vi "FL24 Washer Tool Main.vi"() -> ()   [LabVIEW 2016]
uses:
  Common/LabVIEW GEA2 Toolkit/LabVIEW_GEA2_Toolkit.lvlibp/type defs/Data In.ctl
  Common/LabVIEW GEA2 Toolkit/LabVIEW_GEA2_Toolkit.lvlibp/type defs/Source_Destination.ctl
  Common/LabVIEW GEA2 Toolkit/LabVIEW_GEA2_Toolkit.lvlibp/type defs/Data Type.ctl
  Common/LabVIEW GEA2 Toolkit/LabVIEW_GEA2_Toolkit.lvlibp/type defs/ERD Read Data In.ctl
  Laundry Tool 2.0 Support/type defs2/Select _Graph_Brass.ctl
  Laundry Tool 1.0 Support/type defs/ERD_Graph_All.ctl
  Laundry Tool 1.0 Support/type defs/ERD_Graph.ctl
  Laundry Tool 1.0 Support/type defs/Version.ctl
  Laundry Tool 2.0 Support/type defs2/ERD_Always_Show_FL24_Washer.ctl
  Laundry Tool 1.0 Support/type defs/Fault_Buffer_Status.ctl
  Laundry Tool 2.0 Support/type defs2/Diagnostics_Table.ctl
  Laundry Tool 1.0 Support/type defs/Cycle_Diag_Buffer_Status.ctl
  Laundry Tool 2.0 Support/type defs2/ERD_Data_Loop_Control_Brass.ctl
  Laundry Tool 2.0 Support/type defs2/ERD_Loop_States_Brass.ctl
  Laundry Tool 2.0 Support/type defs2/Error_Command_Brass.ctl
  Laundry Tool 2.0 Support/type defs2/DAQ_States_Brass.ctl
  Common/GExplorer Support/typedefs/GExplorer_Data_Cluster.ctl
  Laundry Tool 1.0 Support/type defs/Cont_Send_States.ctl
  Laundry Tool 2.0 Support/type defs2/Cont_Send_States_Brass.ctl
  Common/LabVIEW GEA2 Toolkit/LabVIEW_GEA2_Toolkit.lvlibp/type defs/Data Out.ctl
  Common/LabVIEW GEA2 Toolkit/LabVIEW_GEA2_Toolkit.lvlibp/type defs/ERD Write Data In.ctl
  Laundry Tool 2.0 Support/type defs2/DAQ_Control_Command_Brass.ctl
  Laundry Tool 2.0 Support/type defs2/ERD_Loop_Control_Command_Brass.ctl
  Laundry Tool 2.0 Support/type defs2/GEA2_Control_Command_Brass.ctl
  <vilib>/DAQmx/read.llb/DAQmx Read (Digital 1D Bool NChan 1Samp 1Line).vi
  <vilib>/DAQmx/read.llb/DAQmx Read (Digital 1D U8 1Chan NSamp).vi
  <vilib>/DAQmx/write.llb/DAQmx Write (Digital Bool 1Line 1Point).vi
  <vilib>/DAQmx/read.llb/DAQmx Read (Counter U32 1Chan 1Samp).vi
  <vilib>/DAQmx/write.llb/DAQmx Write (Analog 1D DBL NChan 1Samp).vi
  <vilib>/DAQmx/write.llb/DAQmx Write (Digital 1D Bool NChan 1Samp 1Line).vi
  Common/LabVIEW GEA2 Toolkit/LabVIEW_GEA2_Toolkit.lvlibp/advanced/GEA2 Message Received Event Handler.vi
  <vilib>/DAQmx/create/channels.llb/DAQmx Create Channel (DO-Digital Output).vi
  <vilib>/DAQmx/create/channels.llb/DAQmx Create Channel (DI-Digital Input).vi
  <vilib>/DAQmx/configure/timing.llb/DAQmx Timing (Sample Clock).vi
  <vilib>/DAQmx/create/channels.llb/DAQmx Create Channel (CO-Pulse Generation-Frequency).vi
  <vilib>/DAQmx/configure/timing.llb/DAQmx Timing (Implicit).vi
  <vilib>/DAQmx/create/channels.llb/DAQmx Create Channel (CI-Count Edges).vi
  <vilib>/DAQmx/create/channels.llb/DAQmx Create Channel (AO-Voltage-Basic).vi
  <vilib>/DAQmx/miscellaneous.llb/DAQmx Fill In Error Info.vi
  C:/Automation/DLLs/PC Dot Net/GeaCommunication.dll
  Common/LabVIEW GEA2 Toolkit/LabVIEW_GEA2_Toolkit.lvlibp
  Automation/Product Specific/Clothes Care/2015 VA Washer/Projects/2015 VA Washer.lvlib
  <resource>/objmgr/daqmx.rc
panel:
  in  "Data ON":bool=TRUE
  out "ERD_Always Show":T1
  in  "Stop":bool
  out "Fault Status":bool
  out "Log Rate (ms)":u32
  in  "Tab Control":T2(tab)
  in  "Filter Data":bool=TRUE
  in  "Start Send":bool
  in  "Cmd":string
  in  "Filter Log":bool
  in  "Msg Rate (ms)":u32=1000 min=50 step=50
  out "CSV File Log Path":path=path "C:/Users/502129737/Desktop/1"
  in  "Clear":bool
  out "GEA2 Log":string
  in  "Board Index":u8 max=0 step=1
  out "Board ID":string="0"
  in  "GEA2 Send":T3={"Source"=228, "Destination"=52, "Command"=0, "Message"=""} {"Command" format="%02x"; "Destination" format="%02x"; "Source" format="%02x"}
  in  "Send Button":bool
  in  "GEA2 Log Length":i32=100000
  in  "Save Log":bool
  out "Version":T4
  in  "GEA Inputs":T5={"Source"=228, "Destination"=52} {"Destination" format="%.0x"; "Source" format="%.0x"}
  in  "Read ERD List":T6[](array[typedef])=[{"ERD Number"=0, "Data Type"=enum."string"}] {"ERD Number" format="%.0x"}
  out "Read ERD Data Out":cluster{"ERD Number":u16, "Data":string}[](array[cluster]) {"ERD Number" format="%.0x"}
  in  "Read ERD":bool
  in  "Write ERD":bool
  in  "Write ERD List":T8(array[cluster])=[{"ERD Number"=0, "Data Type"=enum."string", "Data"=""}] {"ERD Number" format="%.0x"}
  out "All Loads":u16[][](graph)=[[0, 100, 200, 300, 400]]
  in  "ERD Graphing ON":bool
  out "ERD Graph  Ind":T9
  in  "ERD Graph Cntrl":T10={"ERD 3"={"ERD #"=62250, "Data Type"=enum."uint16_t", "Scaler"=32}, "ERD 2"={"ERD #"=62250, "Data Type"=enum."uint16_t", "Scaler"=32}, "ERD 1"={"ERD #"=62250, "Data Type"=enum."uint16_t", "Scaler"=32}} {"ERD 1"."Scaler" min=1; "ERD 1"."ERD #" format="%.0x"; "ERD 2"."Scaler" min=1; "ERD 2"."ERD #" format="%.0x"; "ERD 3"."Scaler" min=1; "ERD 3"."ERD #" format="%.0x"}
  in  "Graphing ON":bool=TRUE
  in  "Select Graph":T12
  out "ERD 3":dbl(graph)
  out "ERD 2":dbl(graph)
  out "ERD 1":dbl(graph)
  in  "Save Fault Log":bool
  in  "Clear Fault Table Buffer":bool
  in  "Clear Fault Seq Buffer":bool
  in  "Fault ON":bool
  out "Fault Table Buffer":string[][](table)
  out "Fault Sequence Buffer":string
  out "Seq Buffer Status":T13
  out "Table Buffer Status":T13
  in  "Save Cycle History Log":bool
  in  "Clear Cycle Buffer":bool
  out "Cycle Buffer Status":T14
  in  "Get Cycle History":bool
  out "Diagnostics Table":T15
  in  "Test Mode":cluster{"Exit":bool, "Enter":bool}
  in  "Lid Lock":cluster{"Lock Lid":bool, "Unlock Lid":bool}
  in  "HE/LE ?":enum16{"HE", "LE"}(ring)
  in  "LL (M - A)":bool=TRUE
  in  "Lid Lock Feedback":bool
  in  "MS (M - A)":bool=TRUE
  out "DAQ Status":string
  out "Drain Pump":bool
  out "Mode Shift":bool
  out "Recirc Pump":bool
  out "Cold Valve":bool
  out "Hot Valve":bool
  out "Spray/Rinse Valve":bool
  out "Fabric SoftValve":bool
  in  "AC Power":bool=TRUE
  in  "Mode Shift FB":bool
  in  "Lid Status":bool=TRUE
  in  "Pressure":dbl(slide) min=0.0 max=5.0 step=0.5 scale=0.0..5.0 scale format="%#_3g"
  in  "Motor Current":dbl(slide)=2.5 min=0.0 max=5.0 step=0.5 scale=0.0..5.0 scale format="%#_3g"
  in  "Turn On DAQ":bool
  out "DAQ On?":bool
  in  "Basket RPM":dbl=1.0 min=1.0 max=800.0 step=5.0
  in  "Temperature":dbl(slide)=2.5 min=0.0 max=5.0 step=0.5 scale=0.0..5.0 scale format="%#_3g"
  out "Triac CW":bool
  out "Traic CCW":bool
  out "CCW":u32
  out "CW":u32
  in  "ERD Read List":T16(array[cluster])=[{"Boolean"=TRUE, "ERD Number"=1, "ERD Name"="Model Number", "Data Type"=enum."string"}, {"Boolean"=TRUE, "ERD Number"=2, "ERD Name"="Serial Number", "Data Type"=enum."string"}, {"Boolean"=TRUE, "ERD Number"=8192, "ERD Name"="Machine Status", "Data Type"=enum."uint8_t"}, {"Boolean"=TRUE, "ERD Number"=8202, "ERD Name"="Cycle Name", "Data Type"=enum."string"}, {"Boolean"=TRUE, "ERD Number"=8213, "ERD Name"="Soil Level", "Data Type"=enum."string"}, {"Boolean"=TRUE, "ERD Number"=142, "ERD Name"="Cycle Count", "Data Type"=enum."uint32_t"}, {"Boolean"=TRUE, "ERD Number"=8193, "ERD Name"="Sub-Cycle", "Data Type"=enum."string"}, {"Boolean"=TRUE, "ERD Number"=141, "ERD Name"="System Runtime", "Data Type"=enum."uint32_t"}, {"Boolean"=TRUE, "ERD Number"=8208, "ERD Name"="Delay Time", "Data Type"=enum."uint16_t"}, {"Boolean"=FALSE, "ERD Number"=256, "ERD Name"="Version", "Data Type"=enum."string"}, {"Boolean"=TRUE, "ERD Number"=70, "ERD Name"="Cycle Time", "Data Type"=enum."uint16_t"}, {"Boolean"=TRUE, "ERD Number"=8206, "ERD Name"="Operating Mode", "Data Type"=enum."string"}, {"Boolean"=TRUE, "ERD Number"=8214, "ERD Name"="Temp Level", "Data Type"=enum."uint8_t"}, {"Boolean"=TRUE, "ERD Number"=8215, "ERD Name"="Spin Level", "Data Type"=enum."uint8_t"}, {"Boolean"=TRUE, "ERD Number"=61440, "ERD Name"="Water Level", "Data Type"=enum."uint8_t"}, {"Boolean"=TRUE, "ERD Number"=8216, "ERD Name"="Rinse Option", "Data Type"=enum."uint8_t"}, {"Boolean"=TRUE, "ERD Number"=8236, "ERD Name"="Basket Speed", "Data Type"=enum."uint16_t"}, {"Boolean"=TRUE, "ERD Number"=61451, "ERD Name"="Loads 2", "Data Type"=enum."uint8_t"}, {"Boolean"=TRUE, "ERD Number"=8210, "ERD Name"="Door Status", "Data Type"=enum."string"}, {"Boolean"=TRUE, "ERD Number"=8211, "ERD Name"="Lock Status", "Data Type"=enum."string"}] {"ERD Number" format="%.0x"}
  out "Error Out":errorcluster
  in  "Error In":errorcluster
  # "Software Version"
  # "UI"
  # "MC"
  # "Must input a valid ERD# and Data Type\nDO NOT Leave Blank \nIf no scaler use value of 01"
  # "Contact:\n\nDerek Hibdon\nderek.hibdon@ge.com"
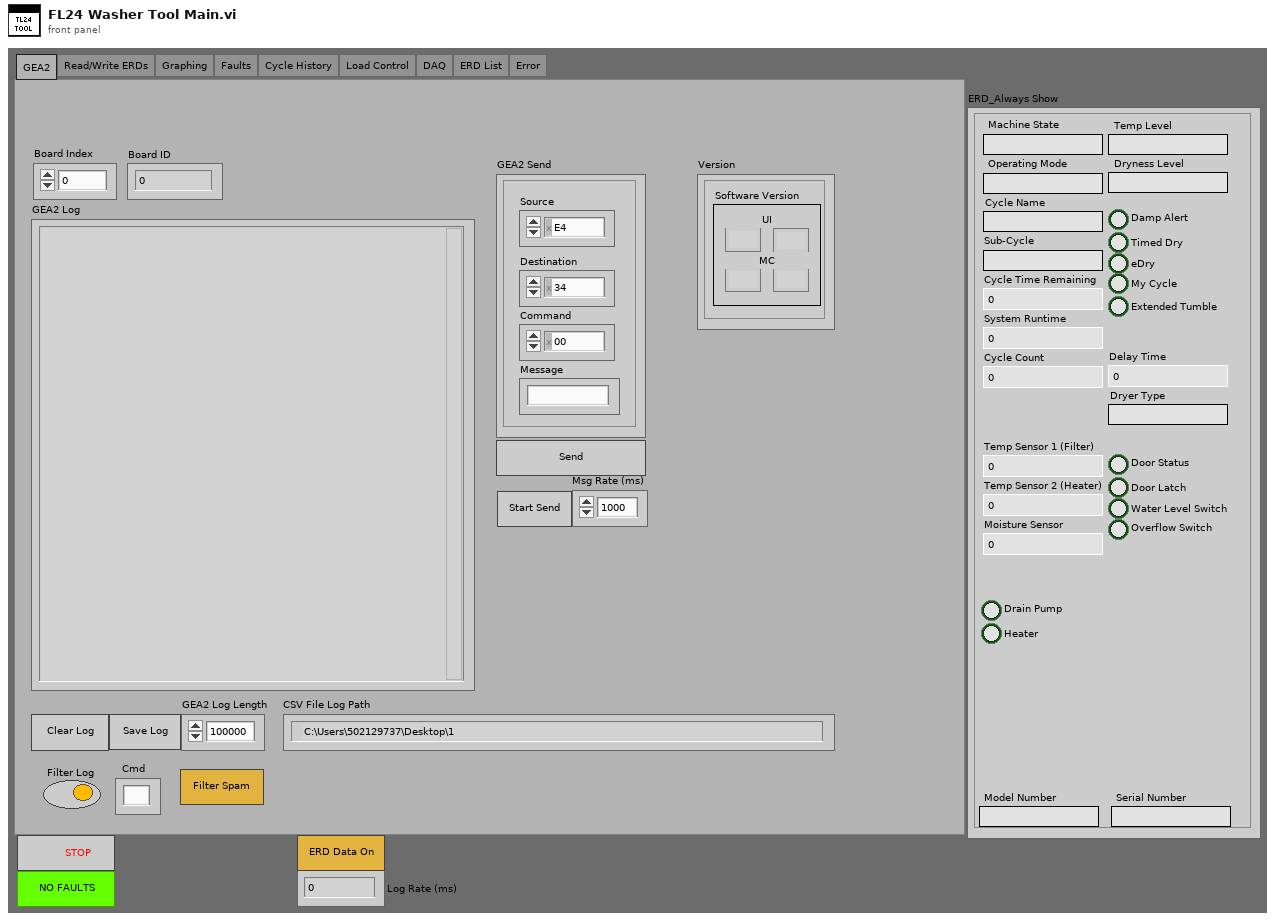
[diagram p1: front panel]
types:
  T1 = typedef "ERD_Always_Show_FL24_Washer.ctl" = cluster{"Machine State":string, "Cycle Count":u32, "Dryness Level":string, "Temp Level":string, "Delay Time":u16, "Sub-Cycle":string, "Cycle Name":string, "Model Number":string, "Serial Number":string, "System Runtime":u32, "Cycle Time Remaining":u16, "Operating Mode":string, "Temp Sensor 1 (Filter)":u16, "Drain Pump":bool, "Water Level Switch":bool, "Overflow Switch":bool, "Door Status":bool, "Door Latch":bool, "Heater":bool, "Temp Sensor 2 (Heater)":u16, "Moisture Sensor":u16, "Dryer Type":string, "eDry":bool, "Damp Alert":bool, "Timed Dry":bool, "My Cycle":bool, "Extended Tumble":bool}
  T2 = enum32{"GEA2", "Read/Write ERDs", "Graphing", "Faults", "Cycle History", "Load Control", "DAQ", "ERD List", "Error"}
  T3 = typedef "LabVIEW_GEA2_Toolkit.lvlibp/Data In.ctl" = cluster{"Source":u8, "Destination":u8, "Command":u8, "Message":string}
  T4 = typedef "Version.ctl" = cluster{"Critical Major":string, "Critical Minor":string, "Non-Critical Minor":string, "Non-Critical Major":string}
  T5 = typedef "LabVIEW_GEA2_Toolkit.lvlibp/Source_Destination.ctl" = cluster{"Source":u8, "Destination":u8}
  T6 = typedef "LabVIEW_GEA2_Toolkit.lvlibp/ERD Read Data In.ctl" = cluster{"ERD Number":u16, "Data Type":T7}
  T7 = typedef "LabVIEW_GEA2_Toolkit.lvlibp/Data Type.ctl" = enum16{"string", "boolean", "uint8_t", "uint16_t", "uint32_t", "uint64_t", "int8_t", "int16_t", "int32_t", "int64_t"}
  T8 = cluster{"ERD Number":u16, "Data Type":T7, "Data":string}[]
  T9 = cluster{"ERD Value 1":dbl, "ERD Value 2":dbl, "ERD Value 3":dbl}
  T10 = typedef "ERD_Graph_All.ctl" = cluster{"ERD 3":T11, "ERD 2":T11, "ERD 1":T11}
  T11 = typedef "ERD_Graph.ctl" = cluster{"ERD #":u16, "Data Type":T7, "Scaler":u32}
  T12 = typedef "Select _Graph_Brass.ctl" = enum16{"All Loads", "ERD 1", "ERD 2", "ERD 3", "Temperature (F)", "Basket Speed (RPM)", "Tub Volume (Gal)", "Pressure (in H2O)", "Current RMS (Amps)"}
  T13 = typedef "Fault_Buffer_Status.ctl" = cluster{"Current Index":u16, "Count":u16, "Overwrite Count":u16}
  T14 = typedef "Cycle_Diag_Buffer_Status.ctl" = cluster{"Current Index":u16, "Count":u16, "Overwrite Count":u16}
  T15 = typedef "Diagnostics_Table.ctl" = string[][]
  T16 = cluster{"Boolean":bool, "ERD Number":u16, "ERD Name":string, "Data Type":enum16{"string", "boolean", "uint8_t", "uint16_t", "uint32_t", "uint64_t"}}[]
  T17 = typedef "Cont_Send_States_Brass.ctl" = enum16{"Run", "Shutdown"}
  T18 = typedef "Cont_Send_States.ctl" = enum16{"Run", "Shutdown"}
  T19 = typedef "GExplorer_Data_Cluster.ctl" = cluster{"Data":variant, "State":enum16{"Add to Log", "Clear", "Shutdown"}}
  T20 = typedef "DAQ_States_Brass.ctl" = enum16{"Wait for Init", "Rename Devices", "Verify Hardware", "Initialize", "Run", "Shutdown", "Exit"}
  T21 = typedef "ERD_Data_Loop_Control_Brass.ctl" = cluster{"Data":variant, "State":T22}
  T22 = typedef "ERD_Loop_States_Brass.ctl" = enum16{"Init", "Build ERD Read List", "Read ERDs", "Update UI", "Update Graphs", "Read Faults", "Log Data", "Pause", "Shutdown"}
  T23 = typedef "Error_Command_Brass.ctl" = enum16{"Initialize", "Handle Errors", "Report Errors"}
  T24 = typedef "LabVIEW_GEA2_Toolkit.lvlibp/ERD Write Data In.ctl" = cluster{"ERD Number":u16, "Data Type":T7, "Data":string}
  T25 = typedef "GEA2_Control_Command_Brass.ctl" = enum16{"Initialize", "Shutdown"}
  T26 = typedef "ERD_Loop_Control_Command_Brass.ctl" = enum16{"Initialize", "Shutdown"}
  T27 = typedef "DAQ_Control_Command_Brass.ctl" = enum16{"Initialize", "Shutdown", "Exit"}
  T28 = enum8{"Enabled", "Disabled", "Disabled and Grayed Out"}
  T29 = typedef "LabVIEW_GEA2_Toolkit.lvlibp/Data Out.ctl" = cluster{"Source":u8, "Destination":u8, "Command":u8, "Length":u8, "CRC":u16, "Message":string}
  T30 = typedef "LabVIEW_GEA2_Toolkit.lvlibp/ERD Read Data Out.ctl" = cluster{"ERD Number":u16, "Data":string}
  T31 = typedef "All_Bundled_Data_Brass.ctl" = cluster{"Version":T4, "ERD_Always Show":T1, "Personality Set":u8, "CSV File String Arrays":T32, "Fault Table Array ":T33}
  T32 = typedef "CSV_File_String_Arrays.ctl" = cluster{"ERD Number Array":string[], "ERD Name Array":string[], "ERD Converted String Data":string[]}
  T33 = typedef "Fault Table Array.ctl" = T34[]
  T34 = typedef "Fault_Table_Info.ctl" = cluster{"Cycle Count":u32, " Runtime (min) ":u32, "Fault Status":string, "Fault ID":string, "Fault Count":u16}
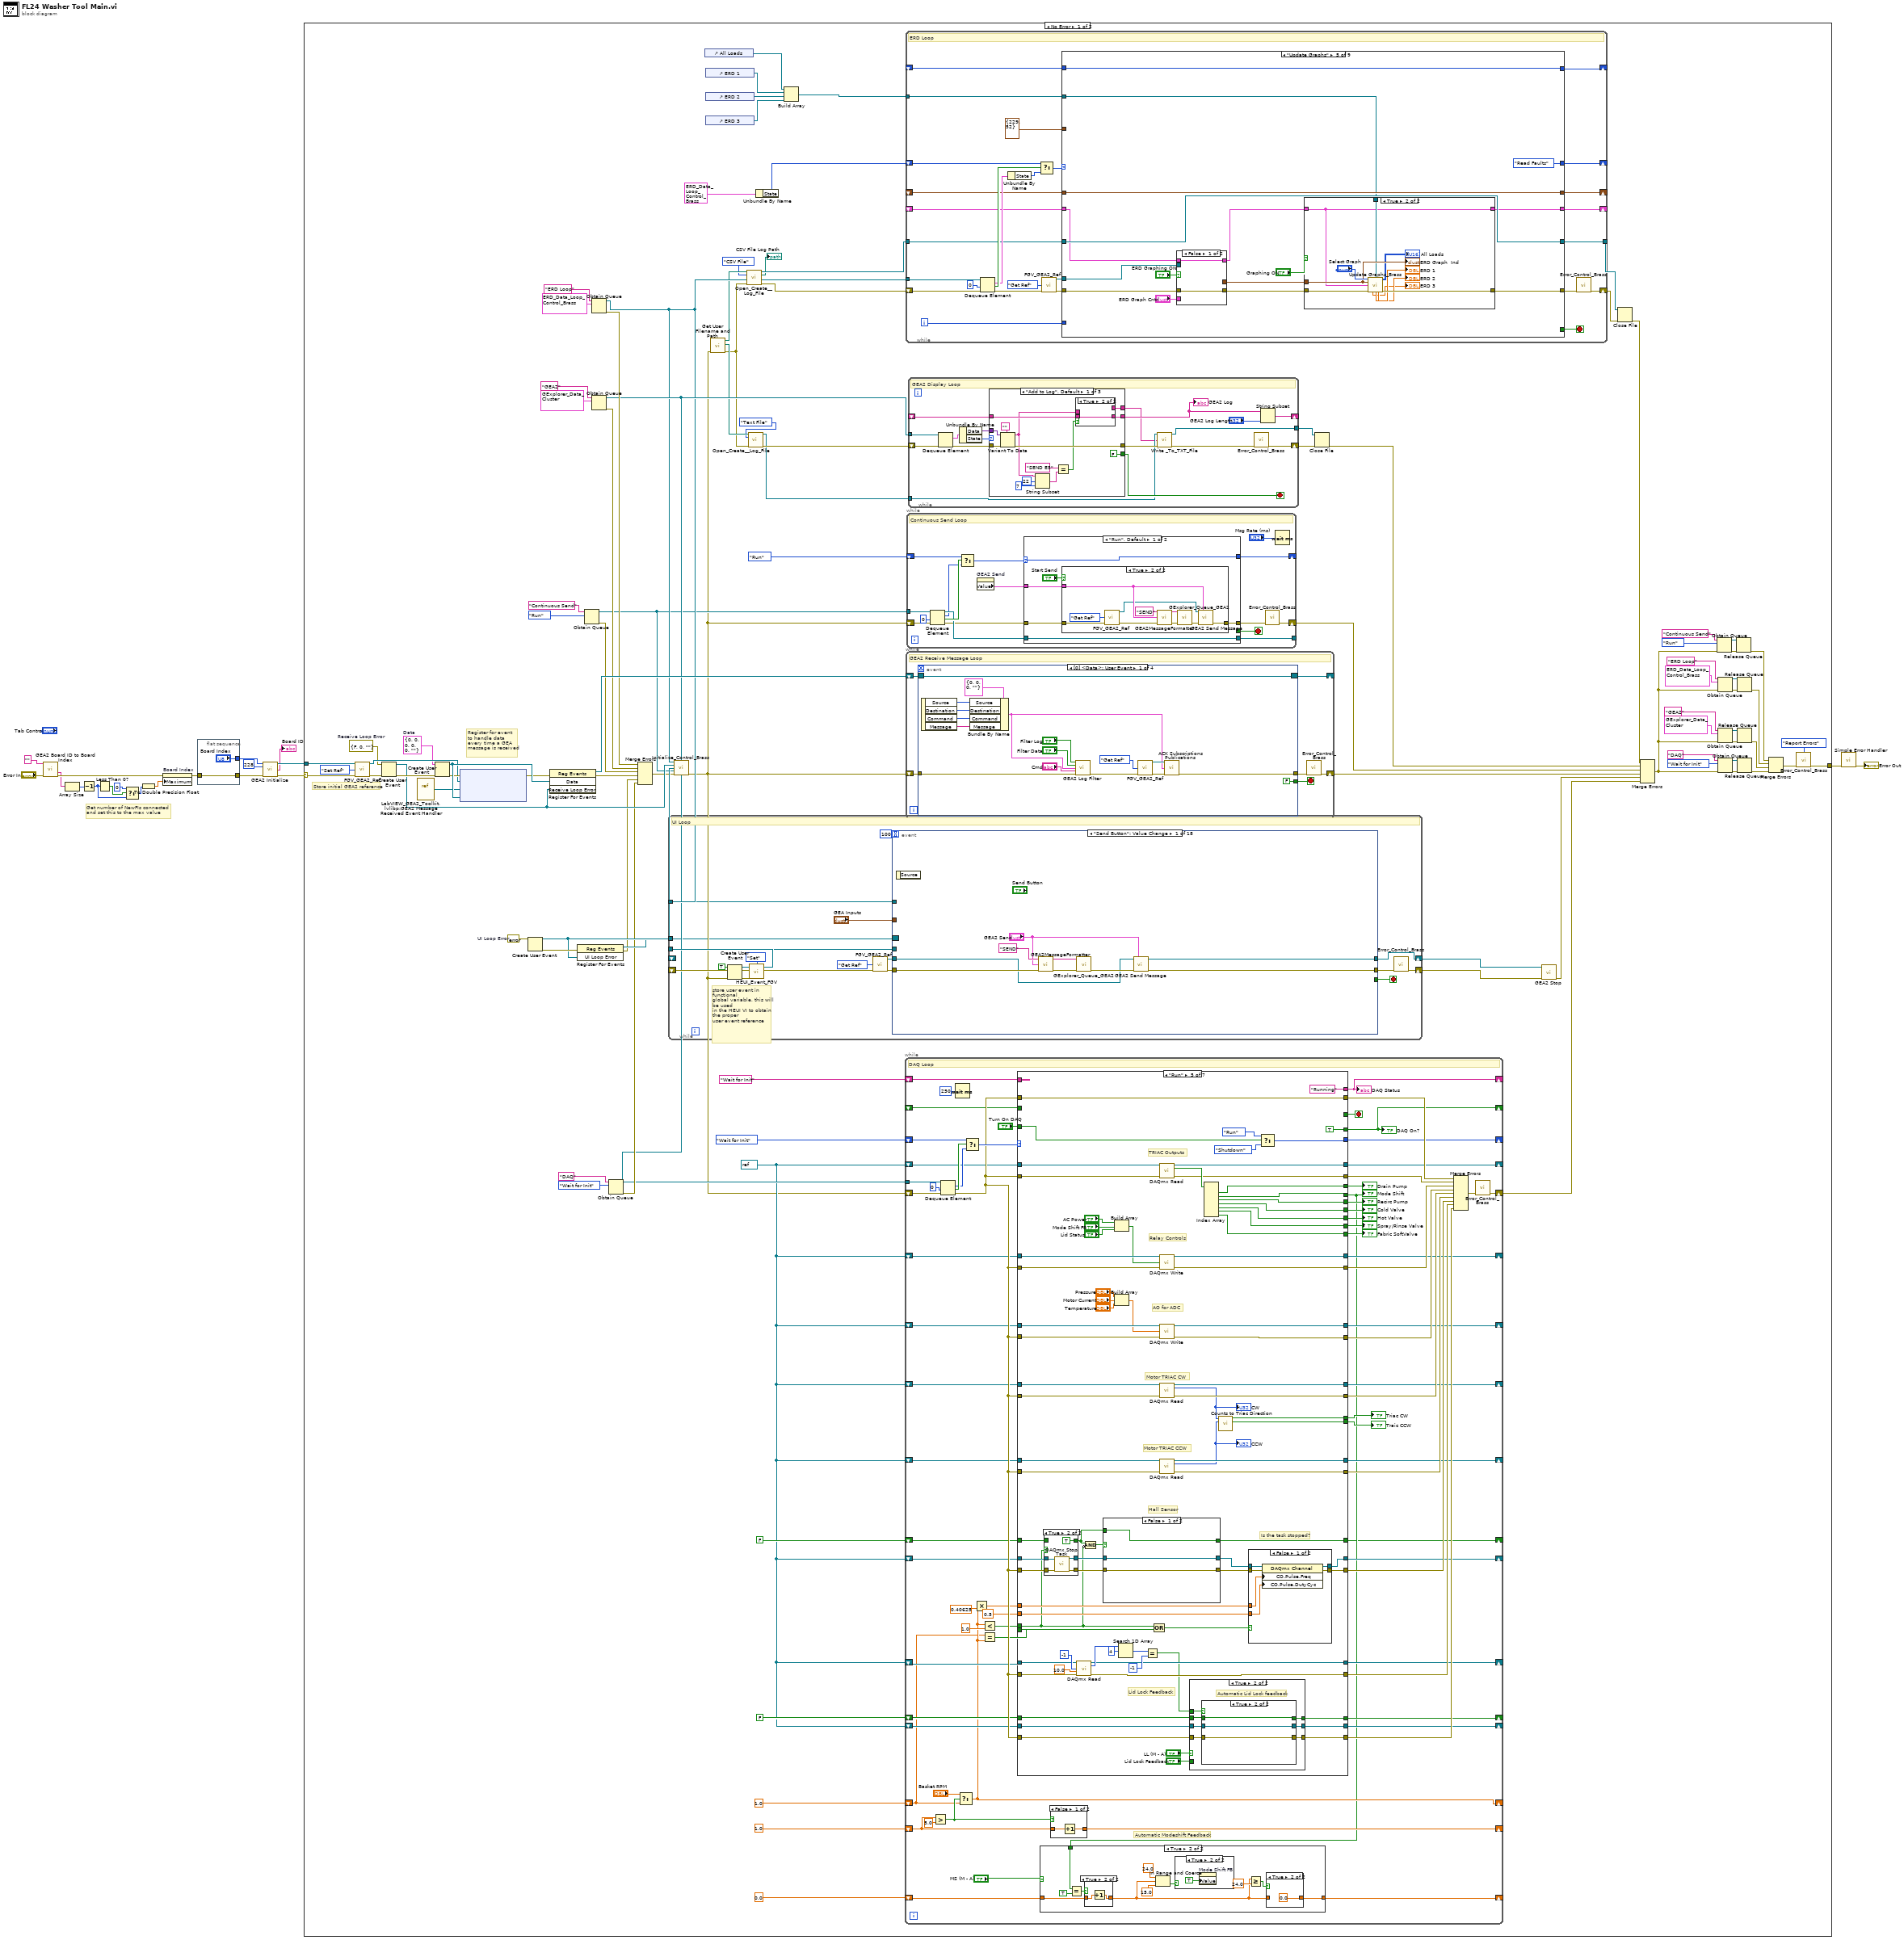
[diagram p0: block diagram]
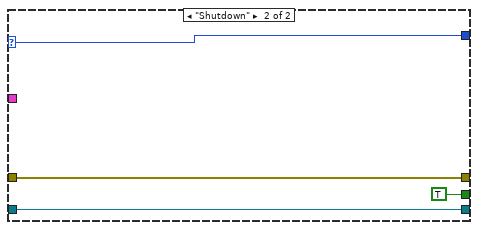
[diagram p3: hidden frame]
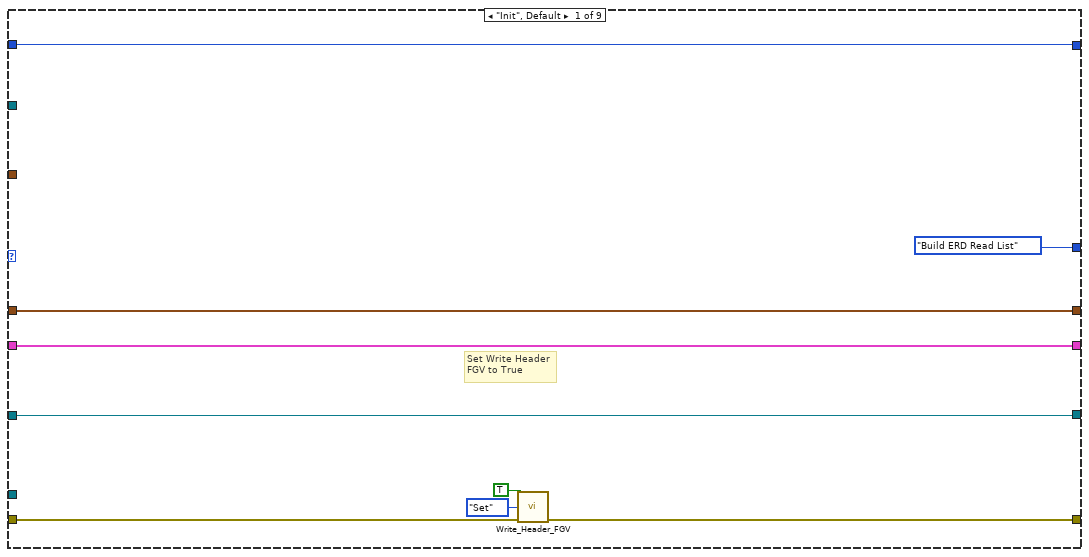
[diagram p4: hidden frame]
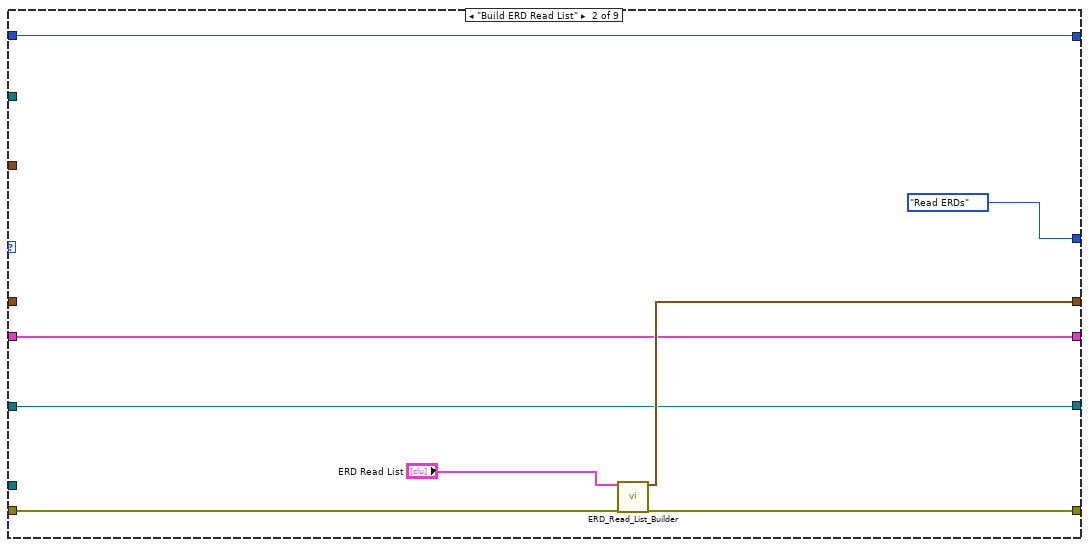
[diagram p5: hidden frame]
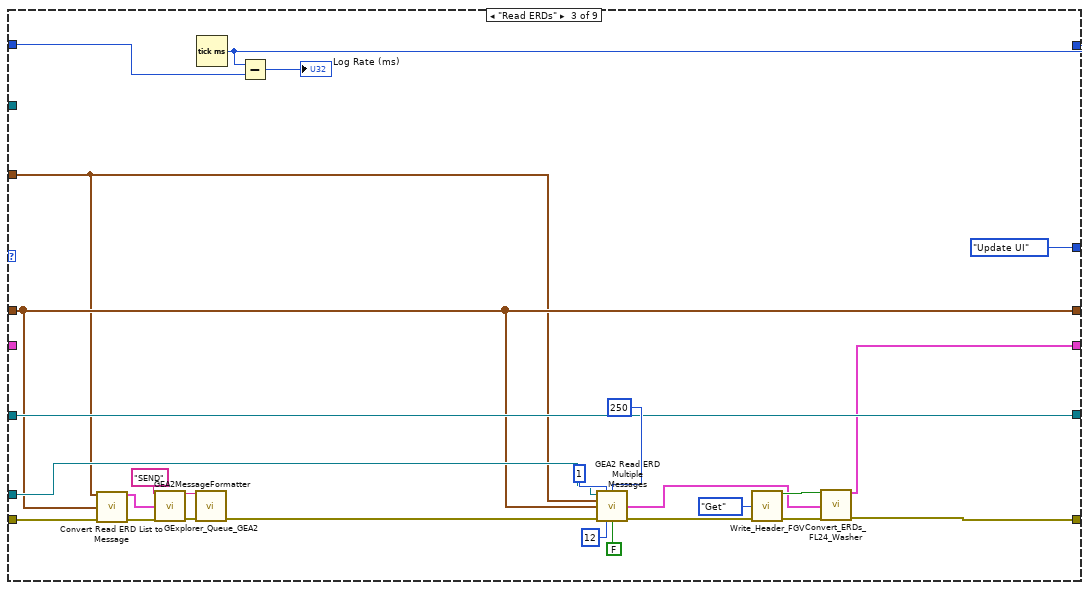
[diagram p6: hidden frame]
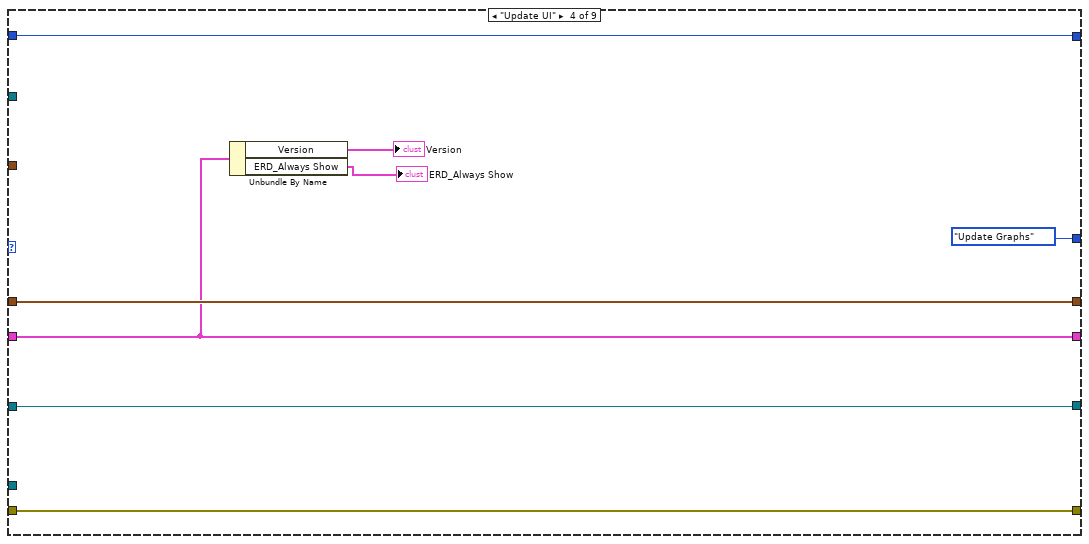
[diagram p7: hidden frame]
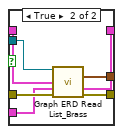
[diagram p9: hidden frame]
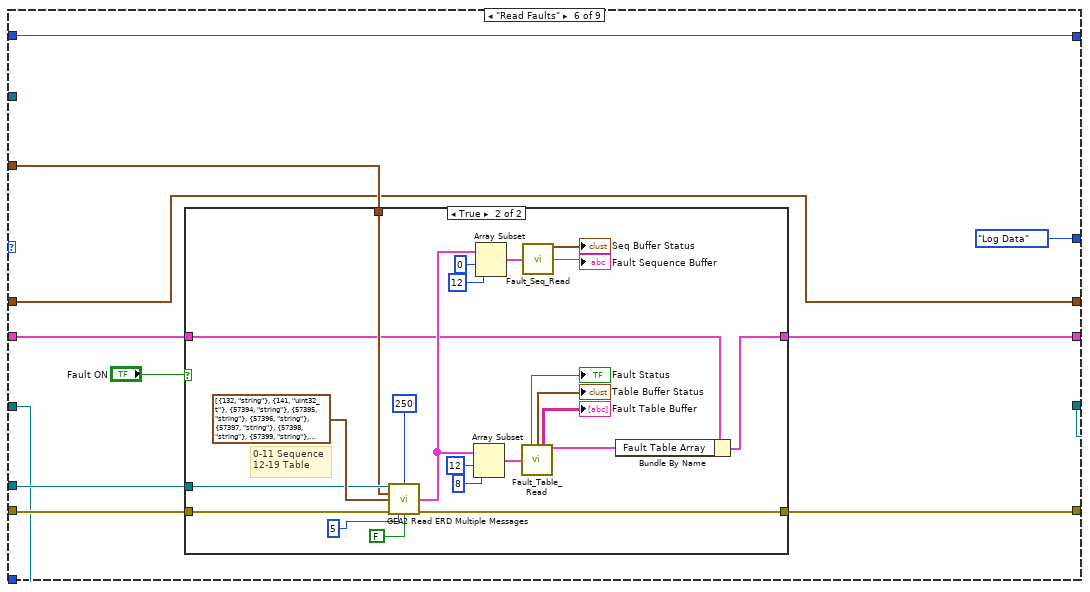
[diagram p10: hidden frame]
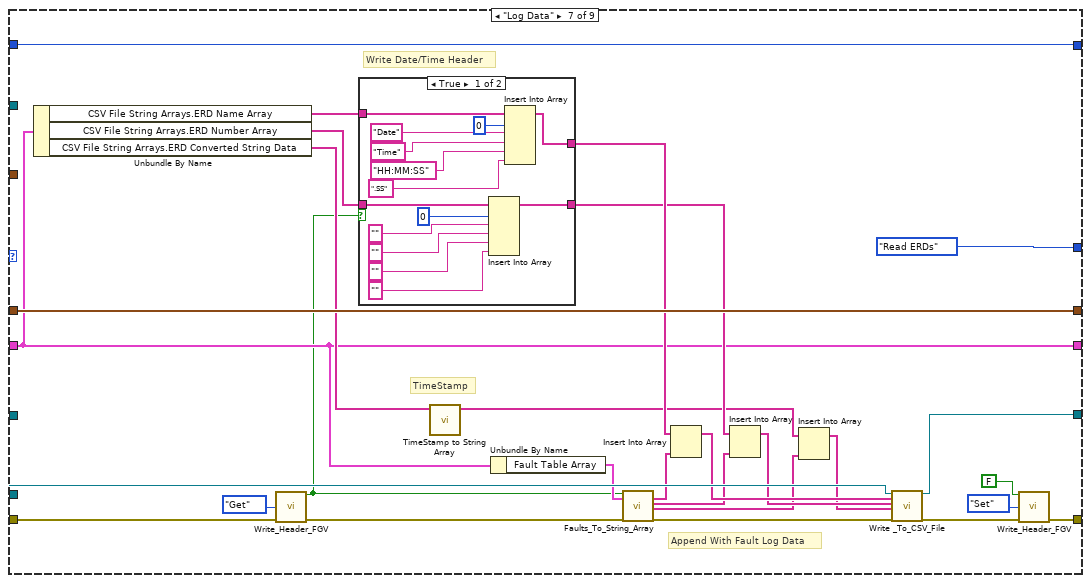
[diagram p12: hidden frame]
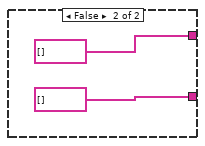
[diagram p13: hidden frame]
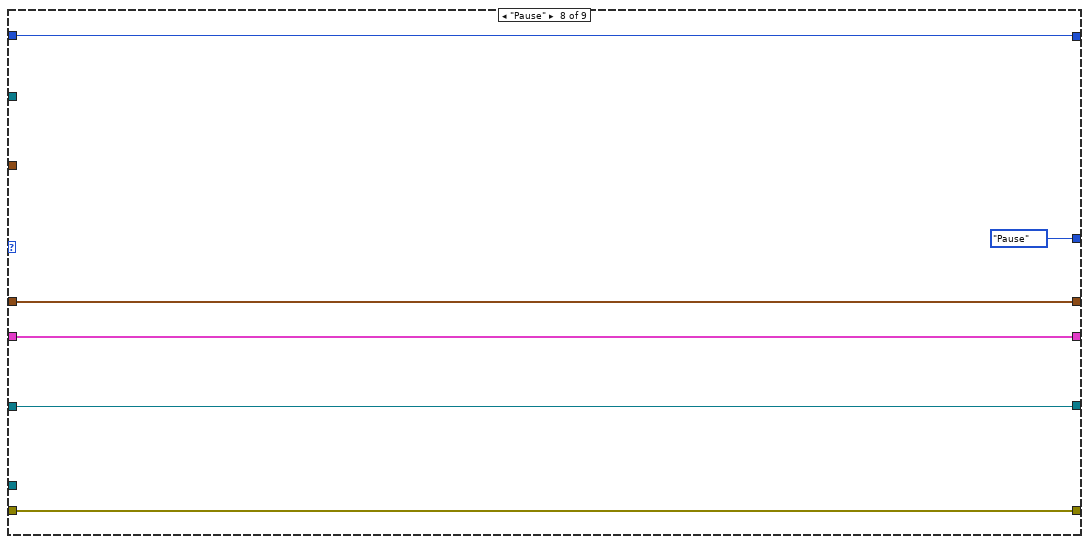
[diagram p14: hidden frame]
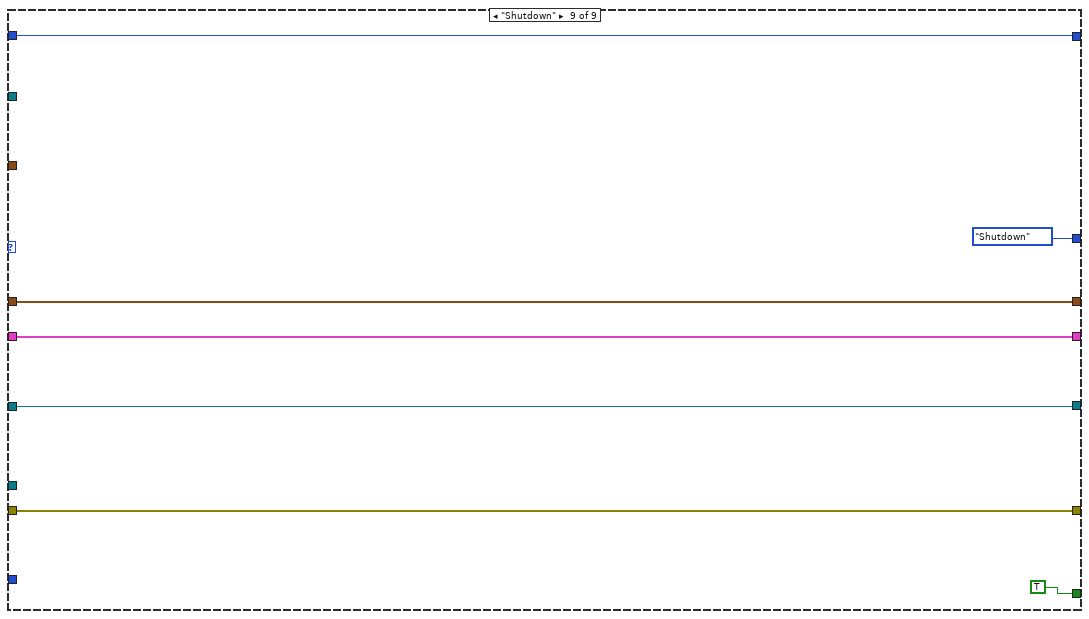
[diagram p15: hidden frame]
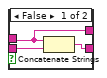
[diagram p16: hidden frame]
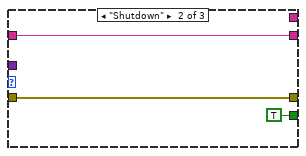
[diagram p17: hidden frame]
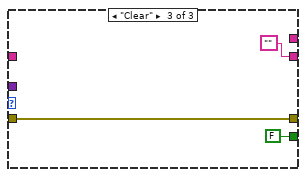
[diagram p18: hidden frame]
diagram:
  # "Get number of NewFIs connected\nand set this to the max value"
  n1 = call "GEA2 Board ID to Board Index.vi"("Board ID"="", "Error In"="Error In") -> ("Boards Found"=w4:string[], "Error Out"=w13:errorcluster)  [unwired: 9 in, 3 out]
  n2 = Array Size(array=w4) -> (size(s)=w9:i32)
  n3 = Decrement(x=w9) -> (x-1=w7:i32)
  n4 = Less Than 0?(x=w7) -> (x < 0?=w8:bool)
  n5 = Select(t=0, s=w8, f=w7) -> (s? t:f=w5:i32)
  n6 = To Double Precision Float(number=w5) -> (double precision float=w3:dbl)
  n7 = property on="Board Index" class="DigNum (strict)"(error in=w13, "Maximum"=w3) -> (error out=w11:errorcluster)  [unwired: 1 in, 1 out]
  n8 = flat-sequence {
    tunnel: ["Board Index"] -> w16
    tunnel: w11 -> [w20]
    tunnel: [w20] -> w10
    frame #0 {
    }
  }
  n9 = call "GEA2 Initialize.vi"("Board Index"=w16, "Source Address"=u8 228, "error in"=w10) -> ("GEA2 Reference Out"=w18:refnum<k24>, "Board ID"=→"Board ID":string, "error out"=w17:errorcluster)  [unwired: 10 in]
  n10 = case shown="No Error" w17 {
    selector: w17 -> [w81 w1347]
    tunnel: w18 -> [w79 _]
    tunnel: [w83 w1347] -> w2
    frame No Error {
      w35 = errorcluster {"status"=FALSE, "code"=0, "source"=""}  # Receive Loop Error
      w36 = T29 {"Source"=0, "Destination"=0, "Command"=0, "Length"=0, "CRC"=0, "Message"=""}  # Data
      w51 = refnum<k21> refnum ("task out")
      w117 = errorcluster {"status"=FALSE, "code"=0, "source"=""}  # UI Loop Error
      # "store user event in functional\nglobal variable, this will be used\nin the HEUI VI to obtain the proper\nuser event reference"
      # "Store initial GEA2 reference"
      # "Register for event\nto handle data\nevery time a GEA\nmessage is received"
      n11 = call "FGV_GEA2_Ref.vi"("GEA2 Reference In"=w79, "Action"=enum16{"Set Ref", "Get Ref"}."Set Ref", "Error In"=w81) -> ("GEA2 Reference Out"=w78:refnum<k24>, "Error Out"=w80:errorcluster)  [unwired: 11 in]
      n12 = Create User Event(user event datatype=w35, error in=w80) -> (user event=w118:refnum<user-event>, error out=w120:errorcluster)
      n13 = vi-ref "LabVIEW_GEA2_Toolkit.lvlibp:GEA2 Message Received Event Handler.vi"() -> (w119:refnum<vi>)
      n14 = Create User Event(user event datatype=w36, error in=w120) -> (user event=w123:refnum<user-event>, error out=w122:errorcluster)
      n15 = node(w122, w78, w119, w123) -> (w121:errorcluster)  [unwired: 1 in, 1 out]
      n16 = Create User Event(user event datatype=w117) -> (user event=w106:refnum<user-event>, error out=w116:errorcluster)  [unwired: 1 in]
      n17 = register-events(error in=w121, w123, w118) -> (reference out=w115:refnum<event-registration>, error out=w88:errorcluster)  [unwired: 1 in]
      n18 = register-events(error in=w116, w106) -> (reference out=w97:refnum<event-registration>, error out=w87:errorcluster)  [unwired: 1 in]
      n19 = Obtain Queue(name (unnamed)="Continuous Send", element data type=Cont_Send_States_Brass."Run" ("State")) -> (queue out=w37:refnum<queue>, error out=w42:errorcluster)  [unwired: 3 in, 1 out]
      n20 = Obtain Queue(name (unnamed)="ERD Loop", element data type=T21 {"Data"=variant, "State"=enum."Read ERDs"} ("Data")) -> (queue out=w66:refnum<queue>, error out=w84:errorcluster)  [unwired: 3 in, 1 out]
      n21 = Obtain Queue(name (unnamed)="GEA2", element data type=T19 {"Data"=variant, "State"=enum."Add to Log"} ("Data")) -> (queue out=w67:refnum<queue>, error out=w89:errorcluster)  [unwired: 3 in, 1 out]
      n22 = Obtain Queue(name (unnamed)="DAQ", element data type=DAQ_States_Brass."Wait for Init" ("States")) -> (queue out=w59:refnum<queue>, error out=w86:errorcluster)  [unwired: 3 in, 1 out]
      n23 = Merge Errors(w84, w89, w42, w88, w87, w86) -> (w85:errorcluster)
      n24 = call "Initialize_Control_Brass.vi"("ERD Loop"=w66, "GEA2"=w67, "Receive Loop"=w118, "UI Loop Error"=w106, "Cont Send"=w37, "Error In"=w85, "DAQ"=w59) -> ("Error Out"=w32:errorcluster)  [unwired: 8 in]
      n25 = control-ref of="All Loads"() -> (w22:refnum<vi>)
      n26 = control-ref of="ERD 1"() -> (w63:refnum<vi>)
      n27 = control-ref of="ERD 2"() -> (w61:refnum<vi>)
      n28 = control-ref of="ERD 3"() -> (w62:refnum<vi>)
      n29 = call "Get User Filename and Path.vi"("error in (no error)"=w32) -> ("error out"=w24:errorcluster, "TXT File Path"=w30:path, "CSV File Path"=w33:path)  [unwired: 8 in]
      n30 = Create User Event(user event datatype=TRUE ("Bool"), error in=w32) -> (user event=w73:refnum<user-event>, error out=w74:errorcluster)
      n31 = call "Open_Create__Log_File.vi"("File Path Control"=w33, "Enum"=enum16{"CSV File", "Text File"}."CSV File", "Error In"=w24) -> ("refnum out"=w64:refnum<file>, "File Path"=→"CSV File Log Path":path, "Error Out"=w76:errorcluster)  [unwired: 10 in]
      n32 = call "Open_Create__Log_File.vi"("File Path Control"=w30, "Enum"=enum16{"CSV File", "Text File"}."Text File", "Error In"=w24) -> ("refnum out"=w29:refnum<file>, "Error Out"=w31:errorcluster)  [unwired: 10 in, 1 out]
      n33 = call "HEUI_Event_FGV.vi"("Event In"=w73, "Action"=enum16{"Get", "Set"}."Set", "Error In"=w74) -> ("Event Out"=w70:refnum<user-event>, "Error Out"=w71:errorcluster)  [unwired: 11 in]
      n34 = while "UI Loop" {
        shift-right: [w1011] -> w125
        shift-left: w71 -> [w1005]
        shift-right: [w1013] -> w124
        shift-left: _ -> [_]
        tunnel: w97 -> [w1012]
        tunnel: w70 -> [w1002]
        tunnel: w66 -> [w1001]
        stop <- w1010 stop-if-true
        # "UI Loop"
        n35 = call "FGV_GEA2_Ref.vi"("Action"=enum16{"Set Ref", "Get Ref"}."Get Ref", "Error In"=w1005) -> ("GEA2 Reference Out"=w1004:refnum<k24>, "Error Out"=w1006:errorcluster)  [unwired: 12 in]
        n36 = event shown="[0] \"Send Button\": Value Change" {
          selector: w1012 -> [_ _ _ _ _ _ _ _ _ _ _ _ _ _ _ _ _ _]
          dyn-events: _ -> [_ _ _ _ _ _ _ _ _ _ _ _ _ _ _ _ _ _]
          timeout: 100 -> [_ _ _ _ _ _ _ _ _ _ _ _ _ _ _ _ _ _]
          tunnel: [w1019 w1029 w1030 w1036 w1050 w1060 w1073 w1080 w1083 w1102 _ _ w1205 w1224 w1238 w1256 w1276 w1287] -> w1009
          tunnel: w1006 -> [w1016 w1026 w1030 w1032 w1047 w1064 w1071 w1078 w1087 w1105 w1120 w1163 w1208 w1230 w1246 w1262 w1277 w1294]
          tunnel: [_ _ _ _ _ _ _ _ _ _ _ _ _ _ _ _ _ TRUE] -> w1010
          tunnel: w1004 -> [w1014 w1028 w1031 w1034 w1048 _ _ _ w1089 w1104 w1119 w1162 w1207 w1229 w1240 w1261 _ w1297]
          tunnel: [w1021 w1028 w1031 w1037 w1049 _ _ _ _ w1103 _ _ w1206 _ _ _ _ w1297] -> w1013
          tunnel: "GEA Inputs" -> [_ _ _ w1035 w1045 _ _ _ w1088 w1106 w1118 w1161 w1209 w1227 w1239 w1263 _ _]
          tunnel: w1002 -> [_ _ _ _ _ _ _ _ _ _ _ _ _ _ _ _ _ _]
          tunnel: w1001 -> [_ _ _ _ _ _ w1069 w1076 _ _ _ _ _ _ _ _ w1274 _]
          event "Send Button": Value Change {
            n37 = event-data() -> ()  [unwired: 1 in, 1 out]
            n38 = call "GEA2MessageFormatter.vi"("Prefix(Send/Recv)"="SEND", "GEA2 Data In"="GEA2 Send", "Error In"=w1016) -> ("Output String"=w1018:string, "Error Out"=w1017:errorcluster)  [unwired: 11 in]
            n39 = call "GExplorer_Queue_GEA2.vi"("Output String"=w1018, "error in (no error)"=w1017) -> ("error out"=w1020:errorcluster)  [unwired: 13 in]
            n40 = call "GEA2 Send Message.vi"("GEA2 Reference In"=w1014, "Input Data"="GEA2 Send", "Error In"=w1020) -> ("GEA2 Reference Out"=w1021:refnum<k24>, "Error Out"=w1019:errorcluster)  [unwired: 11 in]
          }
          event "Clear": Value Change {
            w1023 = T19 {"Data"=variant, "State"=enum."Clear"} ("element")
            n41 = event-data() -> ()  [unwired: 1 in, 6 out]
            n42 = Obtain Queue(name (unnamed)="GEA2", element data type=w1023, error in (no error)=w1026) -> (queue out=w1024:refnum<queue>, error out=w1027:errorcluster)  [unwired: 2 in, 1 out]
            n43 = Enqueue Element(queue=w1024, element=w1023, error in (no error)=w1027) -> (error out=w1029:errorcluster)  [unwired: 1 in, 2 out]
          }
          event Timeout {
            # "Must have timeout case to give GEA2 FGV a chance to update\nthe GEA2 reference. Otherwise, when we receive an event it may\nbe using a reference that is no longer valid."
            n44 = event-data() -> ()  [unwired: 1 in, 3 out]
          }
          event "Write ERD": Value Change {
            n45 = event-data() -> ()  [unwired: 1 in, 1 out]
            n46 = call "Convert Write ERD List to Message.vi"("GEA Inputs"=w1035, "Write ERD List"="Write ERD List", "Error In"=w1032) -> ("GEA Message"=w1041:T3, "Error Out"=w1042:errorcluster)  [unwired: 11 in]
            n47 = call "GEA2MessageFormatter.vi"("Prefix(Send/Recv)"="SEND", "GEA2 Data In"=w1041, "Error In"=w1042) -> ("Output String"=w1043:string, "Error Out"=w1044:errorcluster)  [unwired: 11 in]
            n48 = call "GExplorer_Queue_GEA2.vi"("Output String"=w1043, "error in (no error)"=w1044) -> ("error out"=w1039:errorcluster)  [unwired: 13 in]
            n49 = call "GEA2 Write ERD.vi"("GEA2 Reference In"=w1034, "GEA Inputs"=w1035, "Write ERD List"="Write ERD List", "Error In"=w1039, "Verify ERD Response?"=FALSE) -> ("GEA2 Reference Out"=w1037:refnum<k24>, "Error Out"=w1036:errorcluster)  [unwired: 8 in, 1 out]
          }
          event "Read ERD": Value Change {
            n50 = event-data() -> ()  [unwired: 1 in, 6 out]
            n51 = call "Convert Read ERD List to Message.vi"("GEA Inputs"=w1045, "Read ERD List"="Read ERD List", "Error In"=w1047) -> ("GEA Message"=w1055:T3, "Error Out"=w1046:errorcluster)  [unwired: 11 in]
            n52 = call "GEA2MessageFormatter.vi"("Prefix(Send/Recv)"="SEND", "GEA2 Data In"=w1055, "Error In"=w1046) -> ("Output String"=w1053:string, "Error Out"=w1052:errorcluster)  [unwired: 11 in]
            n53 = call "GExplorer_Queue_GEA2.vi"("Output String"=w1053, "error in (no error)"=w1052) -> ("error out"=w1056:errorcluster)  [unwired: 13 in]
            n54 = call "GEA2 Read ERD.vi"("GEA2 Reference In"=w1048, "GEA Inputs"=w1045, "Read ERD List"="Read ERD List", "Error In"=w1056, "Verify ERD Response?"=FALSE) -> ("GEA2 Reference Out"=w1049:refnum<k24>, "ERD Data Out"=→"Read ERD Data Out":T30[], "Error Out"=w1050:errorcluster)  [unwired: 7 in, 1 out]
          }
          event "Save Log": Value Change {
            n55 = event-data() -> ()  [unwired: 1 in, 6 out]
            n56 = property on="GEA2 Log" class="Str"(error in=w1064) -> (error out=w1066:errorcluster, "Value"=w1065:string)  [unwired: 1 in, 1 out]
            n57 = Write to Text File(prompt (Choose or enter file path)="Choose filename and path to save txt file to ", text=w1065, error in=w1066) -> (refnum out=w1063:refnum<file>, error out=w1062:errorcluster)  [unwired: 1 in, 1 out]
            n58 = Close File(refnum=w1063, error in=w1062) -> (error out=w1061:errorcluster)  [unwired: 1 out]
            n59 = call <vilib>:"Clear Errors.vi"("error in (no error)"=w1061, "specific error code to clear (0: all)"=43) -> ("error out"=w1060:errorcluster)  [unwired: 4 in, 1 out]
          }
          event "ERD Read List": Value Change {
            n60 = event-data() -> ()  [unwired: 1 in, 6 out]
            n61 = Enqueue Element(queue=w1069, element=T21 {"Data"=variant, "State"=enum."Build ERD Read List"}, error in (no error)=w1071) -> (error out=w1070:errorcluster)  [unwired: 1 in, 2 out]
            n62 = call "Write_Header_FGV.vi"("Write Header ? In"=TRUE, "Action"=enum16{"Get", "Set"}."Set", "Error In"=w1070) -> ("Error Out"=w1073:errorcluster)  [unwired: 11 in, 1 out]
          }
          event "Fault ON", "ERD Graphing ON": Value Change {
            n63 = event-data() -> ()  [unwired: 1 in, 6 out]
            n64 = Enqueue Element(queue=w1076, element=T21 {"Data"=variant, "State"=enum."Build ERD Read List"}, error in (no error)=w1078) -> (error out=w1077:errorcluster)  [unwired: 1 in, 2 out]
            n65 = call "Write_Header_FGV.vi"("Write Header ? In"=TRUE, "Action"=enum16{"Get", "Set"}."Set", "Error In"=w1077) -> ("Error Out"=w1080:errorcluster)  [unwired: 11 in, 1 out]
          }
          event "Save Fault Log": Value Change {
            # "0-16 Sequence\n17-27 Table"
            n66 = event-data() -> ()  [unwired: 1 in, 6 out]
            n67 = call "GEA2 Read ERD Multiple Messages.vi"("GEA2 Reference In"=w1089, "Read Timeout (ms)"=u32 250, "GEA Inputs"=w1088, "Read ERD List"=T6[] [{"ERD Number"=132, "Data Type"=enum."string"}, {"ERD Number"=141, "Data Type"=enum."uint32_t"}, {"ERD Number"=57394, "Data Type"=enum."string"}, {"ERD Number"=57395, "Data Type"=enum."string"}, {"ERD Number"=57396, "Data Type"=enum."string"}, {"ERD Number"=57397, "Data Type"=enum."string"}, {"ERD Number"=57398, "Data Type"=enum."string"}, {"ERD Number"=57399, "Data Type"=enum."string"}, {"ERD Number"=57400, "Data Type"=enum."string"}, {"ERD Number"=57401, "Data Type"=enum."string"}, {"ERD Number"=57402, "Data Type"=enum."string"}, {"ERD Number"=57403, "Data Type"=enum."string"}, {"ERD Number"=57404, "Data Type"=enum."string"}, {"ERD Number"=57405, "Data Type"=enum."string"}, {"ERD Number"=57406, "Data Type"=enum."string"}, {"ERD Number"=57407, "Data Type"=enum."string"}, {"ERD Number"=57408, "Data Type"=enum."string"}, {"ERD Number"=129, "Data Type"=enum."string"}, {"ERD Number"=57444, "Data Type"=enum."string"}, {"ERD Number"=57445, "Data Type"=enum."string"}, {"ERD Number"=57446, "Data Type"=enum."string"}, {"ERD Number"=57447, "Data Type"=enum."string"}, {"ERD Number"=57448, "Data Type"=enum."string"}, {"ERD Number"=57449, "Data Type"=enum."string"}, {"ERD Number"=57450, "Data Type"=enum."string"}, {"ERD Number"=57451, "Data Type"=enum."string"}, {"ERD Number"=57452, "Data Type"=enum."string"}, {"ERD Number"=57453, "Data Type"=enum."string"}], "Error In"=w1087, "#ERDs per message"=14 ("#ERDs per message 2"), "Verify ERD Response?"=FALSE) -> ("ERD Data Out"=w1092:T30[], "Error Out"=w1084:errorcluster)  [unwired: 5 in, 2 out]
            n68 = Array Subset(array=w1092, index=17, length=10) -> (w1093:T30[])
            n69 = Array Subset(array=w1092, index=0, length=17) -> (w1091:T30[])
            n70 = call "Fault_Seq_Read.vi"("Seq ERD In"=w1091) -> ("String"=w1086:string)  [unwired: 13 in, 1 out]
            n71 = call "Fault_Table_Read.vi"("ERD Data Out"=w1093) -> ("Fault Table String Out"=w1085:string[][])  [unwired: 11 in, 3 out]
            n72 = call "Fault_Logging.vi"("String"=w1086, "Fault Table String Out"=w1085, "error in (no error)"=w1084) -> ("error out"=w1083:errorcluster)  [unwired: 12 in]
          }
          event "Clear Fault Seq Buffer": Value Change {
            n73 = event-data() -> ()  [unwired: 1 in, 6 out]
            n74 = Bundle By Name(cluster=T24 {"ERD Number"=133, "Data Type"=enum."string", "Data"=""} ("ERD Read Data In"), "Data"="FF") -> (w1115:T24)
            n75 = Build Array(w1115) -> (w1109:T24[])
            n76 = call "Convert Write ERD List to Message.vi"("GEA Inputs"=w1106, "Write ERD List"=w1109, "Error In"=w1105) -> ("GEA Message"=w1111:T3, "Error Out"=w1112:errorcluster)  [unwired: 11 in]
            n77 = call "GEA2MessageFormatter.vi"("Prefix(Send/Recv)"="SEND", "GEA2 Data In"=w1111, "Error In"=w1112) -> ("Output String"=w1113:string, "Error Out"=w1114:errorcluster)  [unwired: 11 in]
            n78 = call "GExplorer_Queue_GEA2.vi"("Output String"=w1113, "error in (no error)"=w1114) -> ("error out"=w1110:errorcluster)  [unwired: 13 in]
            n79 = call "GEA2 Write ERD.vi"("GEA2 Reference In"=w1104, "Read Timeout (ms)"=u32 2000, "GEA Inputs"=w1106, "Write ERD List"=w1109, "Error In"=w1110, "Verify ERD Response?"=FALSE) -> ("GEA2 Reference Out"=w1103:refnum<k24>, "Error Out"=w1102:errorcluster)  [unwired: 7 in, 1 out]
          }
          event "Lid Lock.Lock Lid", "Lid Lock.Unlock Lid": Value Change {
            n80 = event-data() -> ("CtlRef"=w1117:refnum<vi>)  [unwired: 1 in, 5 out]
            n81 = property class="Bool"(reference=w1117, error in=w1120) -> (reference out=w1123:refnum<vi>, error out=w1124:errorcluster, "Label.Text"=w1125:string)
            n82 = Close Reference(reference=w1123, error in (no error)=w1124) -> (error out=w1122:errorcluster)
            n83 = case shown="\"Unlock Lid\", Default" w1125 {
              tunnel: [w1130 w1156] -> _
              tunnel: w1119 -> [w1131 w1155]
              tunnel: w1122 -> [w1132 w1147]
              tunnel: w1118 -> [w1129 w1146]
              tunnel: [w1128 w1145] -> _
              tunnel: T24 {"ERD Number"=61441, "Data Type"=enum."string", "Data"=""} ("ERD Read Data In") -> [w1126 w1143]
              frame "Unlock Lid", Default {
                n84 = Concatenate Strings("00" ("string")) -> (w1142:string)
                n85 = Bundle By Name(cluster=w1126, "Data"=w1142) -> (w1141:T24)
                n86 = Build Array(w1141) -> (w1134:T24[])
                n87 = call "Convert Write ERD List to Message.vi"("GEA Inputs"=w1129, "Write ERD List"=w1134, "Error In"=w1132) -> ("GEA Message"=w1136:T3, "Error Out"=w1137:errorcluster)  [unwired: 11 in]
                n88 = call "GEA2MessageFormatter.vi"("Prefix(Send/Recv)"="SEND", "GEA2 Data In"=w1136, "Error In"=w1137) -> ("Output String"=w1138:string, "Error Out"=w1139:errorcluster)  [unwired: 11 in]
                n89 = call "GExplorer_Queue_GEA2.vi"("Output String"=w1138, "error in (no error)"=w1139) -> ("error out"=w1135:errorcluster)  [unwired: 13 in]
                n90 = call "GEA2 Write ERD.vi"("GEA2 Reference In"=w1131, "GEA Inputs"=w1129, "Write ERD List"=w1134, "Error In"=w1135, "Verify ERD Response?"=FALSE) -> ("GEA2 Reference Out"=w1128:refnum<k24>, "Error Out"=w1130:errorcluster)  [unwired: 8 in, 1 out]
              }
              frame "Lock Lid" {
                n91 = Concatenate Strings("01" ("string")) -> (w1159:string)
                n92 = Bundle By Name(cluster=w1143, "Data"=w1159) -> (w1158:T24)
                n93 = Build Array(w1158) -> (w1149:T24[])
                n94 = call "Convert Write ERD List to Message.vi"("GEA Inputs"=w1146, "Write ERD List"=w1149, "Error In"=w1147) -> ("GEA Message"=w1151:T3, "Error Out"=w1152:errorcluster)  [unwired: 11 in]
                n95 = call "GEA2MessageFormatter.vi"("Prefix(Send/Recv)"="SEND", "GEA2 Data In"=w1151, "Error In"=w1152) -> ("Output String"=w1153:string, "Error Out"=w1154:errorcluster)  [unwired: 11 in]
                n96 = call "GExplorer_Queue_GEA2.vi"("Output String"=w1153, "error in (no error)"=w1154) -> ("error out"=w1150:errorcluster)  [unwired: 13 in]
                n97 = call "GEA2 Write ERD.vi"("GEA2 Reference In"=w1155, "GEA Inputs"=w1146, "Write ERD List"=w1149, "Error In"=w1150, "Verify ERD Response?"=FALSE) -> ("GEA2 Reference Out"=w1145:refnum<k24>, "Error Out"=w1156:errorcluster)  [unwired: 8 in, 1 out]
              }
            }
          }
          event "Test Mode.Exit", "Test Mode.Enter": Value Change {
            n98 = event-data() -> ("CtlRef"=w1160:refnum<vi>)  [unwired: 1 in, 5 out]
            n99 = property class="Bool"(reference=w1160, error in=w1163) -> (reference out=w1166:refnum<vi>, error out=w1167:errorcluster, "Label.Text"=w1168:string)
            n100 = Close Reference(reference=w1166, error in (no error)=w1167) -> (error out=w1165:errorcluster)
            n101 = case shown="\"Exit\"" w1168 {
              tunnel: [w1173 w1199] -> _
              tunnel: w1162 -> [w1174 w1198]
              tunnel: w1165 -> [w1175 w1190]
              tunnel: w1161 -> [w1172 w1189]
              tunnel: [w1171 w1188] -> _
              tunnel: T24 {"ERD Number"=61440, "Data Type"=enum."string", "Data"=""} ("ERD Read Data In") -> [w1169 w1186]
              frame "Enter", Default {
                n102 = Concatenate Strings("01" ("string")) -> (w1185:string)
                n103 = Bundle By Name(cluster=w1169, "Data"=w1185) -> (w1184:T24)
                n104 = Build Array(w1184) -> (w1177:T24[])
                n105 = call "Convert Write ERD List to Message.vi"("GEA Inputs"=w1172, "Write ERD List"=w1177, "Error In"=w1175) -> ("GEA Message"=w1179:T3, "Error Out"=w1180:errorcluster)  [unwired: 11 in]
                n106 = call "GEA2MessageFormatter.vi"("Prefix(Send/Recv)"="SEND", "GEA2 Data In"=w1179, "Error In"=w1180) -> ("Output String"=w1181:string, "Error Out"=w1182:errorcluster)  [unwired: 11 in]
                n107 = call "GExplorer_Queue_GEA2.vi"("Output String"=w1181, "error in (no error)"=w1182) -> ("error out"=w1178:errorcluster)  [unwired: 13 in]
                n108 = call "GEA2 Write ERD.vi"("GEA2 Reference In"=w1174, "GEA Inputs"=w1172, "Write ERD List"=w1177, "Error In"=w1178, "Verify ERD Response?"=FALSE) -> ("GEA2 Reference Out"=w1171:refnum<k24>, "Error Out"=w1173:errorcluster)  [unwired: 8 in, 1 out]
              }
              frame "Exit" {
                n109 = Concatenate Strings("00" ("string")) -> (w1202:string)
                n110 = Bundle By Name(cluster=w1186, "Data"=w1202) -> (w1201:T24)
                n111 = Build Array(w1201) -> (w1192:T24[])
                n112 = call "Convert Write ERD List to Message.vi"("GEA Inputs"=w1189, "Write ERD List"=w1192, "Error In"=w1190) -> ("GEA Message"=w1194:T3, "Error Out"=w1195:errorcluster)  [unwired: 11 in]
                n113 = call "GEA2MessageFormatter.vi"("Prefix(Send/Recv)"="SEND", "GEA2 Data In"=w1194, "Error In"=w1195) -> ("Output String"=w1196:string, "Error Out"=w1197:errorcluster)  [unwired: 11 in]
                n114 = call "GExplorer_Queue_GEA2.vi"("Output String"=w1196, "error in (no error)"=w1197) -> ("error out"=w1193:errorcluster)  [unwired: 13 in]
                n115 = call "GEA2 Write ERD.vi"("GEA2 Reference In"=w1198, "GEA Inputs"=w1189, "Write ERD List"=w1192, "Error In"=w1193, "Verify ERD Response?"=FALSE) -> ("GEA2 Reference Out"=w1188:refnum<k24>, "Error Out"=w1199:errorcluster)  [unwired: 8 in, 1 out]
              }
            }
          }
          event "Clear Fault Table Buffer": Value Change {
            n116 = event-data() -> ()  [unwired: 1 in, 6 out]
            n117 = Bundle By Name(cluster=T24 {"ERD Number"=130, "Data Type"=enum."string", "Data"=""} ("ERD Read Data In"), "Data"="FF") -> (w1218:T24)
            n118 = Build Array(w1218) -> (w1212:T24[])
            n119 = call "Convert Write ERD List to Message.vi"("GEA Inputs"=w1209, "Write ERD List"=w1212, "Error In"=w1208) -> ("GEA Message"=w1214:T3, "Error Out"=w1215:errorcluster)  [unwired: 11 in]
            n120 = call "GEA2MessageFormatter.vi"("Prefix(Send/Recv)"="SEND", "GEA2 Data In"=w1214, "Error In"=w1215) -> ("Output String"=w1216:string, "Error Out"=w1217:errorcluster)  [unwired: 11 in]
            n121 = call "GExplorer_Queue_GEA2.vi"("Output String"=w1216, "error in (no error)"=w1217) -> ("error out"=w1213:errorcluster)  [unwired: 13 in]
            n122 = call "GEA2 Write ERD.vi"("GEA2 Reference In"=w1207, "Read Timeout (ms)"=u32 2000, "GEA Inputs"=w1209, "Write ERD List"=w1212, "Error In"=w1213, "Verify ERD Response?"=FALSE) -> ("GEA2 Reference Out"=w1206:refnum<k24>, "Error Out"=w1205:errorcluster)  [unwired: 7 in, 1 out]
          }
          event "Clear Cycle Buffer": Value Change {
            n123 = event-data() -> ()  [unwired: 1 in, 6 out]
            n124 = Build Array(T24 {"ERD Number"=136, "Data Type"=enum."string", "Data"="FF"} ("ERD Read Data In")) -> (w1232:T24[])
            n125 = call "Convert Write ERD List to Message.vi"("GEA Inputs"=w1227, "Write ERD List"=w1232, "Error In"=w1230) -> ("GEA Message"=w1234:T3, "Error Out"=w1235:errorcluster)  [unwired: 11 in]
            n126 = call "GEA2MessageFormatter.vi"("Prefix(Send/Recv)"="SEND", "GEA2 Data In"=w1234, "Error In"=w1235) -> ("Output String"=w1236:string, "Error Out"=w1237:errorcluster)  [unwired: 11 in]
            n127 = call "GExplorer_Queue_GEA2.vi"("Output String"=w1236, "error in (no error)"=w1237) -> ("error out"=w1233:errorcluster)  [unwired: 13 in]
            n128 = call "GEA2 Write ERD.vi"("GEA2 Reference In"=w1229, "GEA Inputs"=w1227, "Write ERD List"=w1232, "Error In"=w1233) -> ("Error Out"=w1226:errorcluster)  [unwired: 9 in, 2 out]
            n129 = call "Time Delay6"("error in (no error)"=w1226) -> ("error out"=w1221:errorcluster)  [unwired: 10 in]
            n130 = property on="Get Cycle History" class="Bool (strict)"(error in=w1221, "Val(Sgnl)"=TRUE ("Get Cycle History")) -> (error out=w1225:errorcluster)  [unwired: 1 in, 1 out]
            n131 = call "Time Delay7"("error in (no error)"=w1225) -> ("error out"=w1220:errorcluster)  [unwired: 10 in]
            n132 = property on="Get Cycle History" class="Bool (strict)"(error in=w1220, "Val(Sgnl)"=FALSE ("Get Cycle History")) -> (error out=w1224:errorcluster)  [unwired: 1 in, 1 out]
          }
          event "Get Cycle History": Value Change {
            w1244 = T6[] [{"ERD Number"=135, "Data Type"=enum."string"}, {"ERD Number"=57344, "Data Type"=enum."string"}, {"ERD Number"=57345, "Data Type"=enum."string"}, {"ERD Number"=57346, "Data Type"=enum."string"}, {"ERD Number"=57347, "Data Type"=enum."string"}, {"ERD Number"=57348, "Data Type"=enum."string"}, {"ERD Number"=57349, "Data Type"=enum."string"}, {"ERD Number"=57350, "Data Type"=enum."string"}, {"ERD Number"=57351, "Data Type"=enum."string"}, {"ERD Number"=57352, "Data Type"=enum."string"}, {"ERD Number"=57353, "Data Type"=enum."string"}] ("Read ERD List")
            n133 = event-data() -> ()  [unwired: 1 in, 6 out]
            n134 = call "Convert Read ERD List to Message.vi"("GEA Inputs"=w1239, "Read ERD List"=w1244, "Error In"=w1246) -> ("GEA Message"=w1250:T3, "Error Out"=w1251:errorcluster)  [unwired: 11 in]
            n135 = call "GEA2MessageFormatter.vi"("Prefix(Send/Recv)"="SEND", "GEA2 Data In"=w1250, "Error In"=w1251) -> ("Output String"=w1249:string, "Error Out"=w1248:errorcluster)  [unwired: 11 in]
            n136 = call "GExplorer_Queue_GEA2.vi"("Output String"=w1249, "error in (no error)"=w1248) -> ("error out"=w1245:errorcluster)  [unwired: 13 in]
            n137 = call "GEA2 Read ERD Multiple Messages.vi"("GEA2 Reference In"=w1240, "Read Timeout (ms)"=u32 500, "GEA Inputs"=w1239, "Read ERD List"=w1244, "Error In"=w1245, "#ERDs per message"=4, "Verify ERD Response?"=TRUE) -> ("ERD Data Out"=w1252:T30[], "Error Out"=w1243:errorcluster)  [unwired: 5 in, 2 out]
            n138 = call "Cycle_Diag_Table_Read_TL24.vi"("ERD Data In"=w1252, "error in (no error)"=w1243) -> ("Cycle Buffer Status"=→"Cycle Buffer Status":T14, "Diag Cycle String Out"=→"Diagnostics Table":string[][], "error out"=w1238:errorcluster)  [unwired: 10 in, 1 out]
          }
          event "Save Cycle History Log": Value Change {
            w1260 = T6[] [{"ERD Number"=135, "Data Type"=enum."string"}, {"ERD Number"=57344, "Data Type"=enum."string"}, {"ERD Number"=57345, "Data Type"=enum."string"}, {"ERD Number"=57346, "Data Type"=enum."string"}, {"ERD Number"=57347, "Data Type"=enum."string"}, {"ERD Number"=57348, "Data Type"=enum."string"}, {"ERD Number"=57349, "Data Type"=enum."string"}, {"ERD Number"=57350, "Data Type"=enum."string"}, {"ERD Number"=57351, "Data Type"=enum."string"}, {"ERD Number"=57352, "Data Type"=enum."string"}, {"ERD Number"=57353, "Data Type"=enum."string"}] ("Read ERD List")
            n139 = event-data() -> ()  [unwired: 1 in, 6 out]
            n140 = call "Convert Read ERD List to Message.vi"("GEA Inputs"=w1263, "Read ERD List"=w1260, "Error In"=w1262) -> ("GEA Message"=w1269:T3, "Error Out"=w1270:errorcluster)  [unwired: 11 in]
            n141 = call "GEA2MessageFormatter.vi"("Prefix(Send/Recv)"="SEND", "GEA2 Data In"=w1269, "Error In"=w1270) -> ("Output String"=w1268:string, "Error Out"=w1267:errorcluster)  [unwired: 11 in]
            n142 = call "GExplorer_Queue_GEA2.vi"("Output String"=w1268, "error in (no error)"=w1267) -> ("error out"=w1265:errorcluster)  [unwired: 13 in]
            n143 = call "GEA2 Read ERD Multiple Messages.vi"("GEA2 Reference In"=w1261, "Read Timeout (ms)"=u32 500, "GEA Inputs"=w1263, "Read ERD List"=w1260, "Error In"=w1265, "#ERDs per message"=4, "Verify ERD Response?"=TRUE) -> ("ERD Data Out"=w1259:T30[], "Error Out"=w1264:errorcluster)  [unwired: 5 in, 2 out]
            n144 = call "Cycle_Diag_Table_Read_TL24.vi"("ERD Data In"=w1259, "error in (no error)"=w1264) -> ("Diag Cycle String Out"=w1258:string[][], "error out"=w1257:errorcluster)  [unwired: 10 in, 2 out]
            n145 = call "Cycle_History_Logging.vi"("error in (no error)"=w1257, "Diag Cycle String Out"=w1258) -> ("error out"=w1256:errorcluster)  [unwired: 9 in]
          }
          event "Data ON": Value Change {
            n146 = event-data() -> ()  [unwired: 1 in, 6 out]
            n147 = case shown="True" "Data ON" {
              tunnel: w1277 -> [w1280 w1284]
              tunnel: [w1279 w1283] -> w1276
              tunnel: w1274 -> [w1278 w1282]
              frame True {
                n148 = Enqueue Element(queue=w1278, element=T21 {"Data"=variant, "State"=enum."Init"} ("Data"), error in (no error)=w1280) -> (error out=w1279:errorcluster)  [unwired: 1 in, 2 out]
              }
              frame False {
                n149 = Enqueue Element(queue=w1282, element=T21 {"Data"=variant, "State"=enum."Pause"} ("Data"), error in (no error)=w1284) -> (error out=w1283:errorcluster)  [unwired: 1 in, 2 out]
              }
            }
          }
          event "Stop": Value Change; User Event; Panel Close {
            n150 = event-data() -> ()  [unwired: 1 in, 3 out]
            n151 = call "Control_ERD_Loop_Brass.vi"("Command (ERD Loop Control)"=ERD_Loop_Control_Command_Brass."Shutdown", "Error In"=w1294) -> ("Error Out"=w1293:errorcluster)  [unwired: 13 in]
            n152 = call "Control_GEA2_Loop_Brass.vi"("Command (ERD Loop Control)"=GEA2_Control_Command_Brass."Shutdown", "Error In"=w1293) -> ("Error Out"=w1295:errorcluster)  [unwired: 13 in]
            n153 = call "Control_DAQ_Loop_Brass.vi"("Command (DAQ Control)"=DAQ_Control_Command_Brass."Shutdown", "Error In"=w1295) -> ("Error Out"=w1298:errorcluster)  [unwired: 13 in]
            n154 = call "Control_Cont_Send_Brass.vi"("Command (ERD Loop Control)"=GEA2_Control_Command_Brass."Shutdown", "Error In"=w1298) -> ("Error Out"=w1288:errorcluster)  [unwired: 13 in]
            n155 = call "Time Delay8"("error in (no error)"=w1288, "Delay Time (s)"=2.0) -> ("error out"=w1287:errorcluster)  [unwired: 9 in]
          }
        }
        n156 = call "Error_Control_Brass.vi"("Error In"=w1009) -> ("Error Out"=w1011:errorcluster)  [unwired: 14 in]
      }
      n157 = Unbundle By Name(T21 {"Data"=variant, "State"=enum."Init"} ("Data")) -> ("State"=w68:T22)
      n158 = Build Array(w22, w63, w61, w62) -> (w60:refnum<vi>[])
      n159 = while "DAQ Loop" {
        shift-right: [w484] -> w95
        shift-left: w32 -> [w482]
        shift-right: [w461] -> _
        shift-left: DAQ_States_Brass."Wait for Init" ("States") -> [w479]
        shift-right: [w462] -> _
        shift-left: "Wait for Init" ("Report Text") -> [w477]
        tunnel: w59 -> [w478]
        shift-right: [w460] -> _
        shift-left: _ -> [w417]
        shift-right: [w459] -> _
        shift-left: FALSE -> [w458]
        shift-right: [w448] -> _
        shift-left: w51 -> [w447]
        shift-right: [w446] -> _
        shift-left: w51 -> [w445]
        shift-right: [w444] -> _
        shift-left: w51 -> [w443]
        shift-right: [w442] -> _
        shift-left: w51 -> [w441]
        shift-right: [w440] -> _
        shift-left: w51 -> [w439]
        shift-right: [w438] -> _
        shift-left: w51 -> [w437]
        shift-right: [w436] -> _
        shift-left: w51 -> [w435]
        shift-right: [w422] -> _
        shift-left: 1.0 -> [w418]
        shift-right: [w421] -> _
        shift-left: 1.0 -> [w425]
        shift-right: [w420] -> _
        shift-left: 0.0 -> [w424]
        shift-right: [w416] -> _
        shift-left: w51 -> [w415]
        shift-right: [w414] -> _
        shift-left: FALSE -> [w449]
        stop <- w474 stop-if-true
        # "Automatic Modeshift Feedback"
        # "DAQ Loop"
        n160 = Greater?(x=w425, y=5.0 ("x")) -> (0:w427:bool)
        n161 = Dequeue Element(queue=w478, timeout in ms (-1)=0, error in (no error)=w482) -> (element=w480:T20, timed out?=w481:bool, error out=w473:errorcluster)  [unwired: 1 out]
        n162 = Wait (ms)(milliseconds to wait=u32 250) -> ()  [unwired: 1 out]
        n163 = Select(t="Basket RPM", s=w427, f=w418) -> (s? t:f=w422:dbl)
        n164 = Select(t=w479, s=w481, f=w480) -> (s? t:f=w476:T20)
        n165 = Multiply(x=w422, y=0.40625) -> (x*y=w453:dbl)
        n166 = Less?(x=w422, y=1.0) -> (x < y?=w451:bool)
        n167 = Equal?(x=w418, y=w422) -> (x = y?=w450:bool)
        n168 = case shown="\"Run\"" w476 {
          selector: w476 -> [_ _ _ _ _ _ w963]
          tunnel: [_ _ _ w676 w796 _ _] -> w416
          tunnel: [w516 w540 w572 w677 w794 w901 w966] -> w470
          tunnel: w435 -> [w531 w555 w580 _ w793 w895 w912]
          tunnel: [w531 w555 w580 w681 w792 _ _] -> w436
          tunnel: w437 -> [w530 w554 w581 _ w791 w892 w939]
          tunnel: [w530 w554 w581 w685 w790 _ _] -> w438
          tunnel: [w514 w538 w564 w684 w789 w855 w929] -> w468
          tunnel: [w515 w539 w565 w680 w788 w862 w941] -> w469
          tunnel: [w525 DAQ_States_Brass."Verify Hardware" ("t") w577 DAQ_States_Brass."Run" ("t") w766 DAQ_States_Brass."Wait for Init" ("States") w963] -> w461
          tunnel: [FALSE FALSE FALSE TRUE TRUE FALSE FALSE] -> w460
          tunnel: w443 -> [w529 w553 w584 _ w751 w899 w968]
          tunnel: [w511 w535 w561 w673 w785 w848 w926] -> w465
          tunnel: [w529 w553 w584 w674 w786 _ _] -> w444
          tunnel: [w512 w536 w562 w637 w776 w887 w967] -> w466
          tunnel: w441 -> [w528 w552 w583 _ w775 w898 w962]
          tunnel: [w528 w552 w583 w642 w777 _ _] -> w442
          tunnel: [_ _ _ _ _ FALSE TRUE] -> w474
          tunnel: [_ _ _ _ w784 _ _] -> w434
          tunnel: [_ _ _ _ w778 _ _] -> w419
          tunnel: [_ _ _ _ w783 _ _] -> w433
          tunnel: [_ _ _ _ w782 _ _] -> w432
          tunnel: [_ _ _ _ w781 _ _] -> w431
          tunnel: [_ _ _ _ w780 _ _] -> w430
          tunnel: [_ _ _ _ w779 _ _] -> w429
          tunnel: [w513 w537 w563 w634 w774 w885 w960] -> w467
          tunnel: [w527 w551 w582 w631 w772 _ _] -> w440
          tunnel: w439 -> [w527 w551 w582 _ w773 w886 w961]
          tunnel: [_ _ _ _ w771 _ _] -> w457
          tunnel: [_ _ _ _ w770 _ _] -> w456
          tunnel: [w526 w550 w574 "Initialize" ("Report Text") "Running" ("Report Text") "Wait for Init" ("Report Text") "Exit" ("Report Text")] -> w462
          tunnel: w477 -> [w526 w550 _ _ _ _ _]
          tunnel: [w510 w534 w560 w615 w758 w879 w957] -> w464
          tunnel: [w521 w548 w570 w612 w757 _ _] -> w446
          tunnel: [w520 w547 w569 w610 w755 _ _] -> w448
          tunnel: [w509 w533 w559 w609 w756 w878 w904] -> w463
          tunnel: w445 -> [w521 w548 w570 _ w759 w880 w958]
          tunnel: w447 -> [w520 w547 w569 _ w754 w876 w924]
          tunnel: [w508 w532 w558 w589 w753 FALSE FALSE] -> w459
          tunnel: [FALSE FALSE FALSE FALSE w743 FALSE FALSE] -> w414
          tunnel: [w517 w543 w567 w596 w742 w871 w954] -> w471
          tunnel: "Turn On DAQ" -> [w518 _ _ _ w718 _ _]
          tunnel: w473 -> [w516 w540 w566 w598 w741 w870 w953]
          tunnel: w473 -> [w515 w539 w565 w597 w736 w868 w915]
          tunnel: w473 -> [w517 w542 w567 w596 w742 w871 w954]
          tunnel: w473 -> [w514 w538 w564 w595 w734 w853 w938]
          tunnel: w473 -> [w513 w537 w563 w594 w733 w852 w952]
          tunnel: w473 -> [w512 w536 w562 w593 w730 w851 w951]
          tunnel: w473 -> [w511 w535 w561 w592 w729 w850 w950]
          tunnel: w473 -> [w510 w534 w560 w591 w723 w846 w949]
          tunnel: w473 -> [w509 w533 w559 w590 w719 w845 w923]
          tunnel: w458 -> [w508 w532 w558 w589 w722 _ _]
          tunnel: w453 -> [_ _ _ _ w728 _ _]
          tunnel: 0.5 ("Duty Cycle") -> [_ _ _ _ w727 _ _]
          tunnel: w451 -> [_ _ _ _ w725 _ _]
          tunnel: w450 -> [_ _ _ _ w726 _ _]
          tunnel: w449 -> [_ _ _ _ w724 _ _]
          tunnel: w417 -> [_ _ _ _ _ _ w948]
          tunnel: w415 -> [_ _ _ _ w717 w844 w947]
          frame "Wait for Init", Default {
            # "Hall Sensor"
            # "Motor TRIAC CCW"
            # "Motor TRIAC CW"
            # "Relay Controls"
            # "TRIAC Outputs"
            # "AO for ADC"
            n169 = Select(t=DAQ_States_Brass."Rename Devices", s=w518, f=DAQ_States_Brass."Wait for Init" ("States")) -> (s? t:f=w525:T20)
          }
          frame "Rename Devices" {
            # "Hall Sensor"
            # "Motor TRIAC CCW"
            # "Motor TRIAC CW"
            # "Relay Controls"
            # "TRIAC Outputs"
            n170 = case shown="\"LE\"" "HE/LE ?" {
              tunnel: ["VALEW_HE" "VALEW_LE"] -> w544
              frame "HE", Default {
              }
              frame "LE" {
              }
            }
            n171 = call "VALEW_Rename DAQmx Devices.vi"("cDAQ Name"=w544, "Error In"=w542) -> ("Error Out"=w543:errorcluster)  [unwired: 13 in]
          }
          frame "Verify Hardware" {
            n172 = call "DeviceListCheck.vi"("Device List"=string[] ["9481_1", "9435_1", "9435_2", "9401_1", "9269_1"], "Error In"=w566) -> ("Devices Present?"=w571:bool, "Report Text"=w574:string, "Error Out"=w573:errorcluster)  [unwired: 11 in]
            n173 = case shown="False" w571 {
              selector: w571 -> [w586 _]
              tunnel: w573 -> [w587 w588]
              tunnel: [w585 w588] -> w572
              frame False {
                n174 = property on="Turn On DAQ" class="Bool (strict)"(error in=w587, "Value"=w586) -> (error out=w585:errorcluster)  [unwired: 1 in, 1 out]
              }
              frame True {
              }
            }
            n175 = Select(t=DAQ_States_Brass."Initialize" ("f"), s=w571, f=DAQ_States_Brass."Wait for Init") -> (s? t:f=w577:T20)
          }
          frame "Initialize" {
            w603 = 4 items=["verify"=2, "reserve"=4, "commit"=3, "unreserve"=5, "abort"=6] ("action")
            w619 = 10123 items=["Finite Samples"=10178, "Continuous Samples"=10123, "Hardware Timed Single Point"=12522] ("sample mode")
            w622 = 4 items=["verify"=2, "reserve"=4, "commit"=3, "unreserve"=5, "abort"=6] ("action")
            w655 = 4 items=["verify"=2, "reserve"=4, "commit"=3, "unreserve"=5, "abort"=6] ("action")
            w656 = 4 items=["verify"=2, "reserve"=4, "commit"=3, "unreserve"=5, "abort"=6] ("action")
            w670 = 10123 items=["Finite Samples"=10178, "Continuous Samples"=10123, "Hardware Timed Single Point"=12522] ("sample mode")
            w678 = 0 items=["one channel for each line", "one channel for all lines"] ("line grouping")
            w683 = 0 items=["one channel for each line", "one channel for all lines"] ("line grouping")
            w686 = 0.0  # minimum value
            w687 = 5.0  # maximum value
            # "Hall Sensor"
            # "Motor TRIAC CCW"
            # "Motor TRIAC CW"
            # "Relay Controls"
            # "TRIAC Outputs"
            # "AO for ADC"
            n176 = call <vilib>:"DAQmx Create Task.vi"("auto cleanup"=TRUE, "error in"=w592) -> ("task out"=w644:refnum<k21>, "error out"=w645:errorcluster)  [unwired: 12 in]
            n177 = call <vilib>:"DAQmx Create Task.vi"("auto cleanup"=TRUE, "error in"=w591) -> ("task out"=w618:refnum<k21>, "error out"=w617:errorcluster)  [unwired: 12 in]
            n178 = call <vilib>:"DAQmx Create Task.vi"("auto cleanup"=TRUE, "error in"=w594) -> ("task out"=w652:refnum<k21>, "error out"=w653:errorcluster)  [unwired: 12 in]
            n179 = call <vilib>:"DAQmx Create Task.vi"("auto cleanup"=TRUE, "error in"=w593) -> ("task out"=w650:refnum<k21>, "error out"=w651:errorcluster)  [unwired: 12 in]
            n180 = call-poly <vilib>:"DAQmx Create Virtual Channel.vi"("task in"=w644, "counter"=tag "9401_1/ctr2", "error in"=w645) -> ("task out"=w647:refnum<k21>, "error out"=w675:errorcluster)  [unwired: 11 in]
            n181 = call-poly <vilib>:"DAQmx Create Virtual Channel.vi"("task in"=w652, "counter"=tag "9401_1/ctr0", "error in"=w653) -> ("task out"=w665:refnum<k21>, "error out"=w661:errorcluster)  [unwired: 11 in]
            n182 = call-poly <vilib>:"DAQmx Create Virtual Channel.vi"("task in"=w650, "counter"=tag "9401_1/ctr1", "error in"=w651) -> ("task out"=w664:refnum<k21>, "error out"=w663:errorcluster)  [unwired: 11 in]
            n183 = call-poly <vilib>:"DAQmx Create Virtual Channel.vi"("task in"=w618, "lines"=tag "9401_1/port0/line2", "error in"=w617) -> ("task out"=w624:refnum<k21>, "error out"=w625:errorcluster)  [unwired: 11 in]
            n184 = property class="DAQmx Channel"(reference=w647, error in=w675, "CO.Pulse.Term"=tag "/9401_1/PFI4") -> (reference out=w672:refnum<k21>, error out=w671:errorcluster)
            n185 = call-poly <vilib>:"DAQmx Create Virtual Channel.vi"("lines"=tag "9481_1/port0/line3", "error in"=w590) -> ("task out"=w610:refnum<k21>, "error out"=w609:errorcluster)  [unwired: 12 in]
            n186 = property class="DAQmx Channel"(reference=w665, error in=w661, "CI.CountEdges.Term"=tag "/9401_1/PFI0") -> (reference out=w660:refnum<k21>, error out=w659:errorcluster)
            n187 = property class="DAQmx Channel"(reference=w664, error in=w663, "CI.CountEdges.Term"=tag "/9401_1/PFI1") -> (reference out=w658:refnum<k21>, error out=w657:errorcluster)
            n188 = call-poly <vilib>:"DAQmx Create Virtual Channel.vi"("lines"=tag "9481_1/port0/line0:2", "name to assign"="Relay Outputs", "line grouping"=w683, "error in"=w597) -> ("task out"=w681:refnum<k21>, "error out"=w680:errorcluster)  [unwired: 10 in]
            n189 = call-poly <vilib>:"DAQmx Create Virtual Channel.vi"("lines"=tag "9435_1/port0/line0:2, 9435_2/port0/line0:3", "name to assign"="Outputs", "line grouping"=w678, "error in"=w598) -> ("task out"=w676:refnum<k21>, "error out"=w677:errorcluster)  [unwired: 10 in]
            n190 = call-poly <vilib>:"DAQmx Create Virtual Channel.vi"("maximum value"=w687, "minimum value"=w686, "physical channels"=tag "9269_1/ao0:2" ("lines"), "name to assign"="AO for ADC", "error in"=w595) -> ("task out"=w685:refnum<k21>, "error out"=w684:errorcluster)  [unwired: 9 in]
            n191 = call-poly <vilib>:"DAQmx Timing.vi"("task/channels in"=w624, "sample mode"=w619, "rate"=1000.0, "error in"=w625) -> ("task out"=w620:refnum<k21>, "error out"=w621:errorcluster)  [unwired: 10 in]
            n192 = call-poly <vilib>:"DAQmx Timing.vi"("task/channels in"=w672, "sample mode"=w670, "error in"=w671) -> ("task out"=w602:refnum<k21>, "error out"=w599:errorcluster)  [unwired: 11 in]
            n193 = call <vilib>:"DAQmx Control Task.vi"("task/channels in"=w660, "action"=w655, "error in"=w659) -> ("task out"=w633:refnum<k21>, "error out"=w636:errorcluster)  [unwired: 11 in]
            n194 = call <vilib>:"DAQmx Control Task.vi"("task/channels in"=w658, "action"=w656, "error in"=w657) -> ("task out"=w641:refnum<k21>, "error out"=w639:errorcluster)  [unwired: 11 in]
            n195 = call <vilib>:"DAQmx Control Task.vi"("task/channels in"=w602, "action"=w603, "error in"=w599) -> ("task out"=w601:refnum<k21>, "error out"=w600:errorcluster)  [unwired: 11 in]
            n196 = call <vilib>:"DAQmx Control Task.vi"("task/channels in"=w620, "action"=w622, "error in"=w621) -> ("task out"=w613:refnum<k21>, "error out"=w614:errorcluster)  [unwired: 11 in]
            n197 = flat-sequence {
              tunnel: w601 -> [w691]
              tunnel: w600 -> [w690]
              tunnel: w641 -> [w699]
              tunnel: [w699] -> w640
              tunnel: w639 -> [w698]
              tunnel: [w698] -> w638
              tunnel: w636 -> [w697]
              tunnel: [w697] -> w635
              tunnel: w633 -> [w696]
              tunnel: [w696] -> w632
              tunnel: w614 -> [w694]
              tunnel: w613 -> [w695]
              tunnel: [w693] -> w607
              tunnel: [w692] -> w606
              tunnel: [w691] -> w605
              tunnel: [w690] -> w604
              tunnel: [w703] -> w673
              tunnel: [w702] -> w674
              tunnel: [w713] -> w642
              tunnel: w640 -> [w712]
              tunnel: w638 -> [w711]
              tunnel: [w710] -> w637
              tunnel: w635 -> [w709]
              tunnel: [w708] -> w634
              tunnel: w632 -> [w707]
              tunnel: [w706] -> w631
              tunnel: [w705] -> w615
              tunnel: [w704] -> w612
              tunnel: w607 -> [w705]
              tunnel: w606 -> [w704]
              tunnel: w605 -> [w701]
              tunnel: w604 -> [w700]
              frame #0 {
                n198 = call <vilib>:"DAQmx Start Task.vi"("task/channels in"=w695, "error in"=w694) -> ("task out"=w692:refnum<k21>, "error out"=w693:errorcluster)  [unwired: 12 in]
              }
              frame #1 {
                n199 = call <vilib>:"DAQmx Start Task.vi"("task/channels in"=w707, "error in"=w709) -> ("task out"=w706:refnum<k21>, "error out"=w708:errorcluster)  [unwired: 12 in]
                n200 = call <vilib>:"DAQmx Start Task.vi"("task/channels in"=w712, "error in"=w711) -> ("task out"=w713:refnum<k21>, "error out"=w710:errorcluster)  [unwired: 12 in]
                n201 = call <vilib>:"DAQmx Start Task.vi"("task/channels in"=w701, "error in"=w700) -> ("task out"=w702:refnum<k21>, "error out"=w703:errorcluster)  [unwired: 12 in]
              }
            }
          }
          frame "Run" {
            # "Lid Lock Feedback"
            # "Is the task stopped?"
            # "Hall Sensor"
            # "Motor TRIAC CCW"
            # "Motor TRIAC CW"
            # "AO for ADC"
            # "Relay Controls"
            # "TRIAC Outputs"
            n202 = case shown="True" w725 {
              tunnel: w751 -> [w830 w835]
              tunnel: [w830 w834] -> w749
              tunnel: [w829 w833] -> w750
              tunnel: [w828 TRUE] -> w744
              tunnel: w729 -> [w829 w831]
              tunnel: w724 -> [w828 _]
              frame False {
              }
              frame True {
                n203 = call <vilib>:"DAQmx Stop Task.vi"("task/channels in"=w835, "error in"=w831) -> ("task out"=w834:refnum<k21>, "error out"=w833:errorcluster)  [unwired: 12 in]
              }
            }
            n204 = call-poly <vilib>:"DAQmx Read.vi"("task/channels in"=w759, "number of samples per channel"=-1, "timeout"=10.0, "error in"=w723) -> ("task out"=w757:refnum<k21>, "data"=w763:u8[], "error out"=w758:errorcluster)  [unwired: 9 in]
            n205 = Compound Arithmetic op=AND(w744, invert w725) -> (w746:bool)
            n206 = case shown="False" w746 {
              tunnel: w750 -> [w820 w824]
              tunnel: w749 -> [w821 w823]
              tunnel: [w821 w827] -> w748
              tunnel: [w820 w826] -> w747
              tunnel: w744 -> [w819 _]
              tunnel: [w819 FALSE] -> w743
              frame False {
              }
              frame True {
                n207 = call <vilib>:"DAQmx Start Task.vi"("task/channels in"=w823, "error in"=w824) -> ("task out"=w827:refnum<k21>, "error out"=w826:errorcluster)  [unwired: 12 in]
                n208 = Wait (ms)(milliseconds to wait=u32 1200) -> ()  [unwired: 1 out]
              }
            }
            n209 = Build Array("AC Power", "Mode Shift FB", "Lid Status") -> (w737:bool[])
            n210 = Build Array("Pressure", "Motor Current", "Temperature") -> (w735:dbl[])
            n211 = Search 1D Array(1D array=w763, element=u8 4) -> (index of element=w761:i32)  [unwired: 1 in]
            n212 = Equal?(x=w761, y=-1) -> (x = y?=w752:bool)
            n213 = Compound Arithmetic op=OR(w725, w726) -> (w745:bool)
            n214 = call-poly <vilib>:"DAQmx Read.vi"("task/channels in"=w717, "error in"=w741) -> ("task out"=w796:refnum<k21>, "data"=w795:bool[], "error out"=w794:errorcluster)  [unwired: 11 in]
            n215 = call-poly <vilib>:"DAQmx Write.vi"("task/channels in"=w793, "data"=w737, "error in"=w736) -> ("task out"=w792:refnum<k21>, "error out"=w788:errorcluster)  [unwired: 10 in, 1 out]
            n216 = call-poly <vilib>:"DAQmx Write.vi"("task/channels in"=w791, "data"=w735, "error in"=w734) -> ("task out"=w790:refnum<k21>, "error out"=w789:errorcluster)  [unwired: 10 in, 1 out]
            n217 = call-poly <vilib>:"DAQmx Read.vi"("task/channels in"=w773, "error in"=w733) -> ("task out"=w772:refnum<k21>, "data"=w732:u32, "error out"=w774:errorcluster)  [unwired: 11 in]
            "CW" <- w732
            n218 = call-poly <vilib>:"DAQmx Read.vi"("task/channels in"=w775, "error in"=w730) -> ("task out"=w777:refnum<k21>, "data"=w731:u32, "error out"=w776:errorcluster)  [unwired: 11 in]
            "CCW" <- w731
            n219 = case shown="True" "LL (M - A)" {
              tunnel: [w799 w809] -> w756
              tunnel: [w800 w808] -> w755
              tunnel: w754 -> [w802 w807]
              tunnel: [w798 w806] -> w753
              tunnel: w752 -> [_ w805]
              tunnel: "Lid Lock Feedback" -> [w801 _]
              tunnel: w722 -> [w798 w804]
              tunnel: w719 -> [w797 w803]
              frame False {
                n220 = call-poly <vilib>:"DAQmx Write.vi"("task/channels in"=w802, "data"=w801, "error in"=w797) -> ("task out"=w800:refnum<k21>, "error out"=w799:errorcluster)  [unwired: 10 in, 1 out]
              }
              frame True {
                # "Automatic Lid Lock feedback"
                n221 = case shown="True" w805 {
                  tunnel: w807 -> [w815 w818]
                  tunnel: [w814 w817] -> w809
                  tunnel: [w813 w818] -> w808
                  tunnel: [w812 w816] -> w806
                  tunnel: w804 -> [w811 w816]
                  tunnel: w803 -> [w810 w817]
                  frame False {
                    n222 = Not(x=w811) -> (.not. x?=w812:bool)
                    n223 = call-poly <vilib>:"DAQmx Write.vi"("task/channels in"=w815, "data"=w812, "error in"=w810) -> ("task out"=w813:refnum<k21>, "error out"=w814:errorcluster)  [unwired: 10 in, 1 out]
                  }
                  frame True {
                  }
                }
              }
            }
            n224 = Index Array(array=w795) -> (element #1=w784:bool, element #2=w778:bool, element #3=w783:bool, element #4=w782:bool, element #5=w781:bool, element #6=w780:bool, element #7=w779:bool)  [unwired: 7 in]
            n225 = call "Counts to Triac Direction.vi"("CCW ctr"=w731, "CW ctr"=w732) -> ("CW"=w770:bool, "CCW"=w771:bool)  [unwired: 8 in]
            n226 = case shown="False" w745 {
              tunnel: w748 -> [w841 w843]
              tunnel: w747 -> [w840 w842]
              tunnel: [w839 w843] -> w786
              tunnel: [w838 w842] -> w785
              tunnel: w728 -> [w837 _]
              tunnel: w727 -> [w836 _]
              frame False {
                n227 = property class="DAQmx Channel"(reference=w841, error in=w840, "CO.Pulse.Freq"=w837, "CO.Pulse.DutyCyc"=w836) -> (reference out=w839:refnum<k21>, error out=w838:errorcluster)
              }
              frame True {
              }
            }
            n228 = Select(t=DAQ_States_Brass."Run" ("States"), s=w718, f=DAQ_States_Brass."Shutdown" ("States")) -> (s? t:f=w766:T20)
          }
          frame "Shutdown" {
            w884 = 0.0
            w881 = FALSE ("element")
            # "Hall Sensor"
            # "Motor TRIAC CCW"
            # "Motor TRIAC CW"
            # "Relay Controls"
            # "TRIAC Outputs"
            # "AO for ADC"
            n229 = local read "AC Power"() -> (w869:bool)
            n230 = Build Array(w869, w881, w881) -> (w896:bool[])
            n231 = Build Array(w884, w884, w884) -> (w883:dbl[])
            n232 = call-poly <vilib>:"DAQmx Write.vi"("task/channels in"=w895, "data"=w896, "error in"=w868) -> ("task out"=w889:refnum<k21>, "error out"=w890:errorcluster)  [unwired: 10 in, 1 out]
            n233 = call-poly <vilib>:"DAQmx Write.vi"("task/channels in"=w876, "data"=FALSE, "error in"=w845) -> ("task out"=w875:refnum<k21>, "error out"=w874:errorcluster)  [unwired: 10 in, 1 out]
            n234 = call-poly <vilib>:"DAQmx Write.vi"("task/channels in"=w892, "data"=w883, "error in"=w853) -> ("task out"=w894:refnum<k21>, "error out"=w893:errorcluster)  [unwired: 10 in, 1 out]
            n235 = call "Time Delay4"("error in (no error)"=w890, "Delay Time (s)"=2.0) -> ("error out"=w888:errorcluster)  [unwired: 9 in]
            n236 = call <vilib>:"DAQmx Clear Task.vi"("task in"=w880, "error in"=w846) -> ("error out"=w879:errorcluster)  [unwired: 13 in]
            n237 = call <vilib>:"DAQmx Clear Task.vi"("task in"=w844, "error in"=w870) -> ("error out"=w901:errorcluster)  [unwired: 13 in]
            n238 = call <vilib>:"DAQmx Clear Task.vi"("task in"=w889, "error in"=w888) -> ("error out"=w867:errorcluster)  [unwired: 13 in]
            n239 = call <vilib>:"DAQmx Clear Task.vi"("task in"=w894, "error in"=w893) -> ("error out"=w860:errorcluster)  [unwired: 13 in]
            n240 = call <vilib>:"DAQmx Clear Task.vi"("task in"=w886, "error in"=w852) -> ("error out"=w885:errorcluster)  [unwired: 13 in]
            n241 = call <vilib>:"DAQmx Clear Task.vi"("task in"=w898, "error in"=w851) -> ("error out"=w887:errorcluster)  [unwired: 13 in]
            n242 = call <vilib>:"DAQmx Clear Task.vi"("task in"=w899, "error in"=w850) -> ("error out"=w849:errorcluster)  [unwired: 13 in]
            n243 = call <vilib>:"DAQmx Clear Task.vi"("task in"=w875, "error in"=w874) -> ("error out"=w878:errorcluster)  [unwired: 13 in]
            n244 = property on="Motor Current" class="Slide (strict)"(error in=w860, "Value"=2.5 ("Motor Current")) -> (error out=w858:errorcluster)  [unwired: 1 in, 1 out]
            n245 = property on="Turn On DAQ" class="Bool (strict)"(error in=w867, "Value"=FALSE ("Turn On DAQ")) -> (error out=w865:errorcluster)  [unwired: 1 in, 1 out]
            n246 = property on="Basket RPM" class="DigNum (strict)"(error in=w849, "Value"=1.0 ("Basket RPM")) -> (error out=w848:errorcluster)  [unwired: 1 in, 1 out]
            n247 = property on="Temperature" class="Slide (strict)"(error in=w858, "Value"=2.5 ("Temperature")) -> (error out=w856:errorcluster)  [unwired: 1 in, 1 out]
            n248 = property on="Mode Shift FB" class="Bool (strict)"(error in=w865, "Value"=FALSE ("Mode Shift FB")) -> (error out=w863:errorcluster)  [unwired: 1 in, 1 out]
            n249 = property on="Lid Status" class="Bool (strict)"(error in=w863, "Value"=FALSE ("Lid Status")) -> (error out=w862:errorcluster)  [unwired: 1 in, 1 out]
            n250 = property on="Pressure" class="Slide (strict)"(error in=w856, "Value"=0.0 ("Pressure")) -> (error out=w855:errorcluster)  [unwired: 1 in, 1 out]
          }
          frame "Exit" {
            w919 = FALSE ("element")
            w937 = 0.0
            n251 = local read "AC Power"() -> (w920:bool)
            n252 = Build Array(w920, w919, w919) -> (w916:bool[])
            n253 = call-poly <vilib>:"DAQmx Write.vi"("task/channels in"=w912, "data"=w916, "error in"=w915) -> ("task out"=w913:refnum<k21>, "error out"=w918:errorcluster)  [unwired: 10 in, 1 out]
            n254 = Build Array(w937, w937, w937) -> (w940:dbl[])
            n255 = call-poly <vilib>:"DAQmx Write.vi"("task/channels in"=w924, "data"=FALSE, "error in"=w923) -> ("task out"=w922:refnum<k21>, "error out"=w921:errorcluster)  [unwired: 10 in, 1 out]
            n256 = call-poly <vilib>:"DAQmx Write.vi"("task/channels in"=w939, "data"=w940, "error in"=w938) -> ("task out"=w936:refnum<k21>, "error out"=w935:errorcluster)  [unwired: 10 in, 1 out]
            n257 = call "Time Delay"("error in (no error)"=w918, "Delay Time (s)"=2.0) -> ("error out"=w914:errorcluster)  [unwired: 9 in]
            n258 = case shown="True" w948 {
              tunnel: w913 -> [_ w1000]
              tunnel: w968 -> [_ w999]
              tunnel: [w972 w998] -> w927
              tunnel: [w973 w997] -> w967
              tunnel: [w969 w996] -> w907
              tunnel: [w975 w995] -> w910
              tunnel: [w976 w994] -> w966
              tunnel: w962 -> [_ w993]
              tunnel: w961 -> [_ w992]
              tunnel: [w974 w991] -> w960
              tunnel: w958 -> [_ w990]
              tunnel: [w971 w989] -> w957
              tunnel: w922 -> [_ w988]
              tunnel: [w970 w987] -> w905
              tunnel: w953 -> [w976 w986]
              tunnel: w914 -> [w975 w985]
              tunnel: w952 -> [w974 w984]
              tunnel: w951 -> [w973 w983]
              tunnel: w950 -> [w972 w982]
              tunnel: w949 -> [w971 w981]
              tunnel: w921 -> [w970 w980]
              tunnel: w947 -> [_ w979]
              tunnel: w936 -> [_ w978]
              tunnel: w935 -> [w969 w977]
              frame False {
              }
              frame True {
                # "Hall Sensor"
                # "Motor TRIAC CCW"
                # "Motor TRIAC CW"
                # "Relay Controls"
                # "TRIAC Outputs"
                # "AO for ADC"
                n259 = call <vilib>:"DAQmx Clear Task.vi"("task in"=w990, "error in"=w981) -> ("error out"=w989:errorcluster)  [unwired: 13 in]
                n260 = call <vilib>:"DAQmx Clear Task.vi"("task in"=w988, "error in"=w980) -> ("error out"=w987:errorcluster)  [unwired: 13 in]
                n261 = call <vilib>:"DAQmx Clear Task.vi"("task in"=w979, "error in"=w986) -> ("error out"=w994:errorcluster)  [unwired: 13 in]
                n262 = call <vilib>:"DAQmx Clear Task.vi"("task in"=w1000, "error in"=w985) -> ("error out"=w995:errorcluster)  [unwired: 13 in]
                n263 = call <vilib>:"DAQmx Clear Task.vi"("task in"=w978, "error in"=w977) -> ("error out"=w996:errorcluster)  [unwired: 13 in]
                n264 = call <vilib>:"DAQmx Clear Task.vi"("task in"=w992, "error in"=w984) -> ("error out"=w991:errorcluster)  [unwired: 13 in]
                n265 = call <vilib>:"DAQmx Clear Task.vi"("task in"=w993, "error in"=w983) -> ("error out"=w997:errorcluster)  [unwired: 13 in]
                n266 = call <vilib>:"DAQmx Clear Task.vi"("task in"=w999, "error in"=w982) -> ("error out"=w998:errorcluster)  [unwired: 13 in]
              }
            }
            n267 = call <vilib>:"Clear Errors.vi"("error in (no error)"=w907, "specific error code to clear (0: all)"=-200088) -> ("error out"=w906:errorcluster)  [unwired: 4 in, 1 out]
            n268 = call <vilib>:"Clear Errors.vi"("error in (no error)"=w910, "specific error code to clear (0: all)"=-200088) -> ("error out"=w909:errorcluster)  [unwired: 4 in, 1 out]
            n269 = call <vilib>:"Clear Errors.vi"("error in (no error)"=w905, "specific error code to clear (0: all)"=-200088) -> ("error out"=w904:errorcluster)  [unwired: 4 in, 1 out]
            n270 = property on="Turn On DAQ" class="Bool (strict)"(error in=w909, "Value"=FALSE ("Turn On DAQ")) -> (error out=w945:errorcluster)  [unwired: 1 in, 1 out]
            n271 = property on="Motor Current" class="Slide (strict)"(error in=w906, "Value"=2.5 ("Motor Current")) -> (error out=w933:errorcluster)  [unwired: 1 in, 1 out]
            n272 = property on="Basket RPM" class="DigNum (strict)"(error in=w927, "Value"=1.0 ("Basket RPM")) -> (error out=w926:errorcluster)  [unwired: 1 in, 1 out]
            n273 = property on="Mode Shift FB" class="Bool (strict)"(error in=w945, "Value"=FALSE ("Mode Shift FB")) -> (error out=w943:errorcluster)  [unwired: 1 in, 1 out]
            n274 = property on="Temperature" class="Slide (strict)"(error in=w933, "Value"=2.5 ("Temperature")) -> (error out=w931:errorcluster)  [unwired: 1 in, 1 out]
            n275 = property on="Lid Status" class="Bool (strict)"(error in=w943, "Value"=FALSE ("Lid Status")) -> (error out=w941:errorcluster)  [unwired: 1 in, 1 out]
            n276 = property on="Pressure" class="Slide (strict)"(error in=w931, "Value"=0.0 ("Pressure")) -> (error out=w929:errorcluster)  [unwired: 1 in, 1 out]
          }
        }
        "DAQ Status" <- w462
        "DAQ On?" <- w460
        "Triac CW" <- w457
        "Traic CCW" <- w456
        "Cold Valve" <- w432
        "Recirc Pump" <- w433
        "Mode Shift" <- w419
        "Drain Pump" <- w434
        "Fabric SoftValve" <- w429
        "Spray/Rinse Valve" <- w430
        "Hot Valve" <- w431
        n277 = case shown="True" "MS (M - A)" {
          tunnel: w424 -> [w486 w497]
          tunnel: [w486 w496] -> w420
          tunnel: w419 -> [_ w487]
          frame False {
          }
          frame True {
            n278 = Equal?(x=w487, y=TRUE) -> (x = y?=w494:bool)
            n279 = case shown="True" w494 {
              tunnel: w497 -> [w502 w504]
              tunnel: [w502 w503] -> w489
              frame False {
              }
              frame True {
                n280 = Increment(x=w504) -> (x+1=w503:dbl)
              }
            }
            n281 = In Range and Coerce(upper limit=24.0, x=w489, lower limit=15.0) -> (In Range?=w491:bool)  [unwired: 1 out]
            n282 = case shown="True" w491 {
              frame False {
                n283 = property on="Mode Shift FB" class="Bool (strict)"("Value"=FALSE ("Mode Shift FB")) -> ()  [unwired: 2 in, 2 out]
              }
              frame True {
                n284 = property on="Mode Shift FB" class="Bool (strict)"("Value"=TRUE ("Mode Shift FB")) -> ()  [unwired: 2 in, 2 out]
              }
            }
            n285 = Greater Or Equal?(x=w489, y=24.0) -> (x >= y?=w488:bool)
            n286 = case shown="True" w488 {
              tunnel: w489 -> [w498 _]
              tunnel: [w498 0.0] -> w496
              frame False {
              }
              frame True {
              }
            }
          }
        }
        n287 = case shown="False" w427 {
          tunnel: w425 -> [w506 _]
          tunnel: [w505 0.0] -> w421
          frame False {
            n288 = Increment(x=w506) -> (x+1=w505:dbl)
          }
          frame True {
          }
        }
        n289 = Merge Errors(w471, w470, w469, w468, w467, w466, w465, w464, w463) -> (w472:errorcluster)
        n290 = call "Error_Control_Brass.vi"("Error In"=w472) -> ("Error Out"=w484:errorcluster)  [unwired: 14 in]
      }
      n291 = while "Periodic ERD Query Loop" {
        shift-right: [w187] -> w49
        shift-left: w76 -> [w189]
        tunnel: w66 -> [w190]
        shift-right: [w184] -> _
        shift-left: _ -> [w183]
        shift-right: [w178] -> _
        shift-left: w68 -> [w180]
        shift-right: [w173] -> _
        shift-left: _ -> [w172]
        tunnel: w64 -> [w171]
        tunnel: [w170] -> w47
        shift-right: [w169] -> _
        shift-left: _ -> [w168]
        tunnel: w60 -> [w167]
        i -> [w166]
        stop <- w186 stop-if-true
        # "ERD Loop"
        n292 = Dequeue Element(queue=w190, timeout in ms (-1)=0, error in (no error)=w189) -> (element=w175:T21, timed out?=w181:bool, error out=w188:errorcluster)  [unwired: 1 out]
        n293 = Unbundle By Name(w175) -> ("State"=w165:T22)
        n294 = Select(t=w180, s=w181, f=w165) -> (s? t:f=w179:T22)
        n295 = call "FGV_GEA2_Ref.vi"("Action"=enum16{"Set Ref", "Get Ref"}."Get Ref", "Error In"=w188) -> ("GEA2 Reference Out"=w174:refnum<k24>, "Error Out"=w177:errorcluster)  [unwired: 12 in]
        n296 = case shown="\"Update Graphs\"" w179 {
          tunnel: w177 -> [w200 w208 w221 w235 w254 w290 w336 w364 w372]
          tunnel: [w192 w204 w214 w235 w252 w289 w333 w364 w372] -> w185
          tunnel: [_ _ _ _ _ _ _ _ TRUE] -> w186
          tunnel: [w199 w206 w212 w238 w258 w283 w343 w365 w370] -> w184
          tunnel: w183 -> [w199 w206 w233 w238 w258 w283 w343 w365 w370]
          tunnel: T5 {"Source"=229, "Destination"=52} ("GEA Inputs") -> [_ _ w210 _ _ w287 _ _ _]
          tunnel: [ERD_Loop_States_Brass."Build ERD Read List" ("State") ERD_Loop_States_Brass."Read ERDs" ("State") ERD_Loop_States_Brass."Update UI" ("State") ERD_Loop_States_Brass."Update Graphs" ("State") ERD_Loop_States_Brass."Read Faults" ("State") ERD_Loop_States_Brass."Log Data" ("State") ERD_Loop_States_Brass."Read ERDs" ("State") ERD_Loop_States_Brass."Pause" ("State") ERD_Loop_States_Brass."Shutdown" ("State")] -> w178
          tunnel: w174 -> [_ _ w222 _ w247 w288 _ _ _]
          tunnel: [w197 w207 w211 w240 w256 w284 w342 w362 w368] -> w173
          tunnel: w172 -> [w197 _ w211 w240 w256 w284 w342 w362 w368]
          tunnel: w171 -> [w196 w203 w219 w236 w255 w282 w341 w361 w367]
          tunnel: [w196 w203 w219 w236 w255 w282 w340 w361 w367] -> w170
          tunnel: [w195 w202 w213 w237 w246 w285 w319 w360 w366] -> w169
          tunnel: w168 -> [w195 w202 _ w237 w244 w286 w319 w360 w366]
          tunnel: w167 -> [_ _ _ _ w248 _ _ _ _]
          tunnel: w166 -> [_ _ _ _ _ _ _ _ _]
          frame "Init", Default {
            # "Set Write Header\nFGV to True"
            n297 = call "Write_Header_FGV.vi"("Write Header ? In"=TRUE, "Action"=enum16{"Get", "Set"}."Set", "Error In"=w200) -> ("Error Out"=w192:errorcluster)  [unwired: 11 in, 1 out]
          }
          frame "Build ERD Read List" {
            n298 = call "ERD_Read_List_Builder.vi"("Array"="ERD Read List", "Error In"=w208) -> ("Read ERD List"=w207:T6[], "Error Out"=w204:errorcluster)  [unwired: 16 in]
          }
          frame "Read ERDs" {
            n299 = call "Convert Read ERD List to Message.vi"("GEA Inputs"=w210, "Read ERD List"=w211, "Error In"=w221) -> ("GEA Message"=w230:T3, "Error Out"=w231:errorcluster)  [unwired: 11 in]
            n300 = call "GEA2MessageFormatter.vi"("Prefix(Send/Recv)"="SEND", "GEA2 Data In"=w230, "Error In"=w231) -> ("Output String"=w229:string, "Error Out"=w228:errorcluster)  [unwired: 11 in]
            n301 = call "GExplorer_Queue_GEA2.vi"("Output String"=w229, "error in (no error)"=w228) -> ("error out"=w226:errorcluster)  [unwired: 13 in]
            n302 = Tick Count (ms)() -> (millisecond timer value=w212:u32)
            n303 = Subtract(x=w212, y=w233) -> (x-y=→"Log Rate (ms)":u32)
            n304 = call "GEA2 Read ERD Multiple Messages.vi"("GEA2 Reference In"=w222, "Retry Count"=1, "Read Timeout (ms)"=u32 250, "GEA Inputs"=w210, "Read ERD List"=w211, "Error In"=w226, "#ERDs per message"=12, "Verify ERD Response?"=FALSE) -> ("ERD Data Out"=w209:T30[], "Error Out"=w218:errorcluster)  [unwired: 4 in, 2 out]
            n305 = call "Write_Header_FGV.vi"("Action"=enum16{"Get", "Set"}."Get", "Error In"=w218) -> ("Write Header ? Out"=w215:bool, "Error Out"=w217:errorcluster)  [unwired: 12 in]
            n306 = call "Convert_ERDs_FL24_Washer.vi"("New Header?"=w215, "Array"=w209, "Error In"=w217) -> ("All_ERD_Data_Bundled_Brass"=w213:T31, "Error Out"=w214:errorcluster)  [unwired: 11 in]
          }
          frame "Update UI" {
            n307 = Unbundle By Name(w237) -> ("Version"=→"Version":T4, "ERD_Always Show"=→"ERD_Always Show":T1)
          }
          frame "Update Graphs" {
            n308 = case shown="False" "ERD Graphing ON" {
              tunnel: w254 -> [w272 w279]
              tunnel: [w272 w278] -> w253
              tunnel: "ERD Graph Cntrl" -> [_ w277]
              tunnel: [_ w276] -> w249
              tunnel: w247 -> [_ w275]
              tunnel: w244 -> [w271 w274]
              tunnel: [w271 w273] -> w243
              frame False {
              }
              frame True {
                n309 = call "Graph ERD Read List_Brass.vi"("GEA2 Reference In"=w275, "All_Bundled_Data_Brass"=w274, "ERD Graph Cntrl"=w277, "Error In"=w279) -> ("ERD Graph  Ind"=w276:T9, "All_Bundled_Data_Brass 2"=w273:T31, "Error Out"=w278:errorcluster)  [unwired: 8 in, 1 out]
              }
            }
            n310 = case shown="True" "Graphing ON" {
              tunnel: w253 -> [w259 w270]
              tunnel: [w259 w269] -> w252
              tunnel: w249 -> [_ w267]
              tunnel: w248 -> [_ w262]
              tunnel: w243 -> [w260 w261]
              tunnel: [w260 w261] -> w246
              frame False {
              }
              frame True {
                n311 = call "Update Graphs_Brass.vi"("Select Graph"="Select Graph", "appended array"=w262, "ERD Graph  Ind 2"=w267, "All_Bundled_Data_Brass"=w261, "Error In"=w270) -> ("All Loads"=→"All Loads":u16[][], "ERD 3"=→"ERD 3":dbl, "ERD 2"=→"ERD 2":dbl, "ERD 1"=→"ERD 1":dbl, "Error Out"=w269:errorcluster)  [unwired: 6 in]
                "ERD Graph  Ind" <- w267
              }
            }
          }
          frame "Read Faults" {
            n312 = case shown="True" "Fault ON" {
              tunnel: w290 -> [w291 w299]
              tunnel: [w291 w298] -> w289
              tunnel: w288 -> [_ w297]
              tunnel: w287 -> [_ w296]
              tunnel: w286 -> [w292 w295]
              tunnel: [w292 w294] -> w285
              frame False {
              }
              frame True {
                # "0-11 Sequence\n12-19 Table"
                n313 = call "GEA2 Read ERD Multiple Messages.vi"("GEA2 Reference In"=w297, "Read Timeout (ms)"=u32 250 ("Read Timeout (ms) 2"), "GEA Inputs"=w296, "Read ERD List"=T6[] [{"ERD Number"=132, "Data Type"=enum."string"}, {"ERD Number"=141, "Data Type"=enum."uint32_t"}, {"ERD Number"=57394, "Data Type"=enum."string"}, {"ERD Number"=57395, "Data Type"=enum."string"}, {"ERD Number"=57396, "Data Type"=enum."string"}, {"ERD Number"=57397, "Data Type"=enum."string"}, {"ERD Number"=57398, "Data Type"=enum."string"}, {"ERD Number"=57399, "Data Type"=enum."string"}, {"ERD Number"=57400, "Data Type"=enum."string"}, {"ERD Number"=57401, "Data Type"=enum."string"}, {"ERD Number"=57402, "Data Type"=enum."string"}, {"ERD Number"=57403, "Data Type"=enum."string"}, {"ERD Number"=129, "Data Type"=enum."string"}, {"ERD Number"=57444, "Data Type"=enum."string"}, {"ERD Number"=57445, "Data Type"=enum."string"}, {"ERD Number"=57446, "Data Type"=enum."string"}, {"ERD Number"=57447, "Data Type"=enum."string"}, {"ERD Number"=57448, "Data Type"=enum."string"}, {"ERD Number"=57449, "Data Type"=enum."string"}, {"ERD Number"=57450, "Data Type"=enum."string"}], "Error In"=w299, "#ERDs per message"=5 ("#ERDs per message 2"), "Verify ERD Response?"=FALSE) -> ("ERD Data Out"=w304:T30[], "Error Out"=w298:errorcluster)  [unwired: 5 in, 2 out]
                n314 = Array Subset(array=w304, index=12, length=8) -> (w305:T30[])
                n315 = Array Subset(array=w304, index=0, length=12) -> (w303:T30[])
                n316 = call "Fault_Table_Read.vi"("ERD Data Out"=w305) -> ("Fault Set?"=→"Fault Status":bool, "Table Buffer Status"=→"Table Buffer Status":T13, "Fault Table String Out"=→"Fault Table Buffer":string[][], "Fault Table Array Out"=w293:T33)  [unwired: 11 in]
                n317 = call "Fault_Seq_Read.vi"("Seq ERD In"=w303) -> ("Seq Buffer Status"=→"Seq Buffer Status":T13, "String"=→"Fault Sequence Buffer":string)  [unwired: 13 in]
                n318 = Bundle By Name(cluster=w295, "Fault Table Array"=w293) -> (w294:T31)
              }
            }
          }
          frame "Log Data" {
            # "TimeStamp"
            # "Append With Fault Log Data"
            # "Write Date/Time Header"
            n319 = Unbundle By Name(w319) -> ("CSV File String Arrays.ERD Name Array"=w339:string[], "CSV File String Arrays.ERD Number Array"=w338:string[], "CSV File String Arrays.ERD Converted String Data"=w331:string[])
            n320 = call "Write_Header_FGV.vi"("Action"=enum16{"Get", "Set"}."Get", "Error In"=w336) -> ("Write Header ? Out"=w317:bool, "Error Out"=w330:errorcluster)  [unwired: 12 in]
            n321 = case shown="True" w317 {
              tunnel: w339 -> [w352 _]
              tunnel: [w354 string[] [] ("ERD Name Array")] -> w329
              tunnel: w338 -> [w353 _]
              tunnel: [w357 string[] [] ("ERD Number Array")] -> w327
              frame True {
                n322 = Insert Into Array(array=w353, index=0, new element #1="", new element #2="", new element #3="", new element #4="") -> (w357:string[])
                n323 = Insert Into Array(array=w352, index=0, new element #1="Date", new element #2="Time", new element #3="HH:MM:SS", new element #4=".SS" ("new element/subarray")) -> (w354:string[])
              }
              frame False {
              }
            }
            n324 = call "TimeStamp to String Array.vi"("String Array In"=w331) -> ("String Array Out"=w325:string[])  [unwired: 10 in]
            n325 = Unbundle By Name(w319) -> ("Fault Table Array"=w318:T33)
            n326 = call "Faults_To_String_Array.vi"("Write Header ?"=w317, "Fault Table Entry"=w318, "Error In"=w330) -> ("Fault Header String Array"=w324:string[], "Fault ERD Number String Array"=w323:string[], "Fault Data String Array"=w322:string[], "Error Out"=w320:errorcluster)  [unwired: 13 in]
            n327 = Insert Into Array(array=w329, new element=w324) -> (w328:string[])  [unwired: 1 in]
            n328 = Insert Into Array(array=w327, new element=w323) -> (w326:string[])  [unwired: 1 in]
            n329 = Insert Into Array(array=w325, new element=w322) -> (w321:string[])  [unwired: 1 in]
            n330 = call "Write _To_CSV_File.vi"("Refnum In"=w341, "String Array 1"=w328, "String Array 2"=w326, "String Array 3"=w321, "Error In"=w320) -> ("Refnum Out"=w340:refnum<file>, "Error Out"=w334:errorcluster)  [unwired: 12 in, 1 out]
            n331 = call "Write_Header_FGV.vi"("Write Header ? In"=FALSE, "Action"=enum16{"Get", "Set"}."Set", "Error In"=w334) -> ("Error Out"=w333:errorcluster)  [unwired: 11 in, 1 out]
          }
          frame "Pause" {
          }
          frame "Shutdown" {
          }
        }
        n332 = call "Error_Control_Brass.vi"("Error In"=w185) -> ("Error Out"=w187:errorcluster)  [unwired: 14 in]
      }
      n333 = while "GEA2 Receive Message Loop" {
        shift-right: [w1302] -> w126
        shift-left: w32 -> [w1303]
        shift-right: [w1299] -> _
        shift-left: w115 -> [w1304]
        stop <- w1301 stop-if-true
        # "GEA2 Receive Message Loop"
        n334 = event shown="[0] <Data>: User Event" {
          selector: w1304 -> [w1320 w1322 w1338 w1344]
          dyn-events: [w1320 w1322 w1333 w1344] -> w1299
          timeout: _ -> [_ _ _ _]
          tunnel: w1303 -> [w1319 w1324 w1341 w1346]
          tunnel: [w1307 w1324 w1326 w1346] -> w1300
          tunnel: [FALSE TRUE _ TRUE] -> w1301
          event User Event {
            n335 = event-data() -> ("Source"=w1314:u8, "Destination"=w1313:u8, "Command"=w1312:u8, "Message"=w1311:string)  [unwired: 1 in]
            n336 = Bundle By Name(cluster=T3 {"Source"=0, "Destination"=0, "Command"=0, "Message"=""} ("GEA2 Msg"), "Source"=w1314, "Destination"=w1313, "Command"=w1312, "Message"=w1311) -> (w1305:T3)
            n337 = call "GEA2 Log Filter.vi"("Filter Log"="Filter Log", "Filter Data"="Filter Data", "GEA2 Msg"=w1305, "Cmd to Filter"="Cmd", "error in (no error)"=w1319) -> ("error out"=w1308:errorcluster)  [unwired: 10 in]
            n338 = call "FGV_GEA2_Ref.vi"("Action"=enum16{"Set Ref", "Get Ref"}."Get Ref", "Error In"=w1308) -> ("GEA2 Reference Out"=w1306:refnum<k24>, "Error Out"=w1309:errorcluster)  [unwired: 12 in]
            n339 = call "ACK Subscriptions Publications.vi"("GEA2 Reference In"=w1306, "GEA2 Msg"=w1305, "error in (no error)"=w1309) -> ("error out"=w1307:errorcluster)  [unwired: 11 in, 1 out]
          }
          event User Event {
            n340 = event-data() -> ()  [unwired: 1 in, 1 out]
          }
          event "Board Index": Value Change {
            # "Stop old GEA2\nbus reference"
            # "Allow other references a chance\nto begin using new reference"
            # "Store new GEA2 bus reference"
            # "Update event registration\nand initialize new GEA2 bus"
            # "Get the previous GEA2\nbus ref, but don't stop it\nuntil we update the FGV\nwith the new GEA2 ref"
            n341 = event-data() -> ("NewVal"=w1337:u8)  [unwired: 1 in]
            n342 = property on="Board Index" class="DigNum (strict)"(error in=w1341, "DisabledEnum"=T28."Disabled and Grayed Out" ("Disabled")) -> (error out=w1342:errorcluster)  [unwired: 1 in, 1 out]
            n343 = call "FGV_GEA2_Ref.vi"("Action"=enum16{"Set Ref", "Get Ref"}."Get Ref", "Error In"=w1342) -> ("GEA2 Reference Out"=w1325:refnum<k24>, "Error Out"=w1339:errorcluster)  [unwired: 12 in]
            n344 = call "GEA2_Reregister.vi"("Board Index"=w1337, "Event Registration In"=w1338, "Error In"=w1339) -> ("GEA2 Reference Out"=w1331:refnum<k24>, "Board ID"=w1334:string, "Event Registration Out"=w1333:refnum<event-registration>, "Error Out"=w1335:errorcluster)  [unwired: 9 in]
            n345 = property on="Board Index" class="DigNum (strict)"(error in=w1335, "DisabledEnum"=T28."Enabled" ("Disabled")) -> (error out=w1332:errorcluster)  [unwired: 1 in, 1 out]
            n346 = local write "Board ID"(w1334) -> ()
            n347 = call "FGV_GEA2_Ref.vi"("GEA2 Reference In"=w1331, "Action"=enum16{"Set Ref", "Get Ref"}."Set Ref", "Error In"=w1332) -> ("Error Out"=w1328:errorcluster)  [unwired: 11 in, 1 out]
            n348 = call "Time Delay"("error in (no error)"=w1328, "Delay Time (s)"=3.0) -> ("error out"=w1327:errorcluster)  [unwired: 9 in]
            n349 = call "GEA2 Stop.vi"("GEA2 Reference In"=w1325, "Error In"=w1327) -> ("Error Out"=w1326:errorcluster)  [unwired: 13 in]
          }
          event "Stop": Value Change {
            n350 = event-data() -> ()  [unwired: 1 in, 6 out]
          }
        }
        n351 = call "Error_Control_Brass.vi"("Error In"=w1300) -> ("Error Out"=w1302:errorcluster)  [unwired: 14 in]
      }
      n352 = while "Continuous Send Loop" {
        shift-right: [w140] -> _
        shift-left: Cont_Send_States."Run" ("State") -> [w139]
        tunnel: w37 -> [w141]
        tunnel: [w134] -> _
        shift-right: [w132] -> w41
        shift-left: w32 -> [w143]
        stop <- w142 stop-if-true
        # "Continuous Send Loop"
        n353 = Dequeue Element(queue=w141, timeout in ms (-1)=0, error in (no error)=w143) -> (queue out=w135:refnum<queue>, element=w128:T17, timed out?=w136:bool, error out=w131:errorcluster)
        n354 = Select(t=w139, s=w136, f=w128) -> (s? t:f=w138:T17)
        n355 = property on="GEA2 Send" class="Clust (strict)"() -> ("Value"=w130:T3)  [unwired: 2 in, 2 out]
        n356 = case shown="\"Run\", Default" w138 {
          selector: w138 -> [w147 w162]
          tunnel: w131 -> [w149 w164]
          tunnel: [w148 w164] -> w133
          tunnel: [_ TRUE] -> w142
          tunnel: [w147 w162] -> w140
          tunnel: w135 -> [w146 w161]
          tunnel: [w146 w161] -> w134
          tunnel: w130 -> [w145 _]
          frame "Run", Default {
            n357 = case shown="True" "Start Send" {
              tunnel: w149 -> [w150 w153]
              tunnel: [w150 w157] -> w148
              tunnel: w145 -> [_ w155]
              frame False {
              }
              frame True {
                n358 = call "FGV_GEA2_Ref.vi"("Action"=enum16{"Set Ref", "Get Ref"}."Get Ref", "Error In"=w153) -> ("GEA2 Reference Out"=w151:refnum<k24>, "Error Out"=w152:errorcluster)  [unwired: 12 in]
                n359 = call "GEA2MessageFormatter.vi"("Prefix(Send/Recv)"="SEND", "GEA2 Data In"=w155, "Error In"=w152) -> ("Output String"=w156:string, "Error Out"=w160:errorcluster)  [unwired: 11 in]
                n360 = call "GExplorer_Queue_GEA2.vi"("Output String"=w156, "error in (no error)"=w160) -> ("error out"=w158:errorcluster)  [unwired: 13 in]
                n361 = call "GEA2 Send Message.vi"("GEA2 Reference In"=w151, "Input Data"=w155, "Error In"=w158) -> ("Error Out"=w157:errorcluster)  [unwired: 11 in, 1 out]
              }
            }
          }
          frame "Shutdown" {
          }
        }
        n362 = call "Error_Control_Brass.vi"("Error In"=w133) -> ("Error Out"=w132:errorcluster)  [unwired: 14 in]
        n363 = Wait (ms)(milliseconds to wait="Msg Rate (ms)") -> ()  [unwired: 1 out]
      }
      n364 = while "GEA2 Display Loop" {
        tunnel: w67 -> [w382]
        shift-right: [w379] -> _
        shift-left: _ -> [w385]
        shift-right: [w381] -> w96
        shift-left: w31 -> [w389]
        tunnel: w29 -> [w375]
        tunnel: [w373] -> w27
        stop <- w383 stop-if-true
        # "GEA2 Display Loop"
        n365 = Dequeue Element(queue=w382, error in (no error)=w389) -> (element=w388:T19, error out=w384:errorcluster)  [unwired: 1 in, 2 out]
        n366 = Unbundle By Name(w388) -> ("Data"=w386:variant, "State"=w387:enum16{"Add to Log", "Clear", "Shutdown"})
        n367 = case shown="\"Add to Log\", Default" w387 {
          tunnel: w386 -> [w400 _ _]
          tunnel: w385 -> [w403 w408 _]
          tunnel: [w402 w408 ""] -> w380
          tunnel: w384 -> [w401 w409 w413]
          tunnel: [w398 w409 w413] -> w376
          tunnel: [FALSE TRUE FALSE] -> w383
          tunnel: [w390 _ _] -> w374
          frame "Add to Log", Default {
            n368 = Variant To Data(error in=w401, type="", Variant=w400) -> (data=w392:string, error out=w398:errorcluster)
            n369 = String Subset(string=w392, offset (0)=22, length (rest)=7 ("length (rest)")) -> (substring=w393:string)
            n370 = Equal?(x="SEND E5", y=w393) -> (x = y?=w391:bool)
            n371 = case shown="True" w391 {
              tunnel: w403 -> [w406 w407]
              tunnel: [w405 w407] -> w402
              tunnel: w392 -> [w404 _]
              tunnel: [w404 _] -> w390
              frame False {
                n372 = Concatenate Strings(w404, w406) -> (w405:string)
              }
              frame True {
              }
            }
          }
          frame "Shutdown" {
          }
          frame "Clear" {
          }
        }
        "GEA2 Log" <- w380
        n373 = call "Write _To_TXT_File.vi"("refnum"=w375, "text"=w374, "error in"=w376) -> ("refnum out"=w373:refnum<file>, "error out"=w377:errorcluster)  [unwired: 10 in, 1 out]
        n374 = call "Error_Control_Brass.vi"("Error In"=w377) -> ("Error Out"=w381:errorcluster)  [unwired: 14 in]
        n375 = String Subset(string=w380, length (rest)="GEA2 Log Length") -> (substring=w379:string)  [unwired: 1 in]
      }
      n376 = Close File(refnum=w27, error in=w96) -> (error out=w28:errorcluster)  [unwired: 1 out]
      n377 = call "GEA2 Stop.vi"("GEA2 Reference In"=w124, "Error In"=w125) -> ("Error Out"=w108:errorcluster)  [unwired: 13 in]
      n378 = Close File(refnum=w47, error in=w49) -> (error out=w48:errorcluster)  [unwired: 1 out]
      n379 = Merge Errors(w48, w28, w41, w126, w108, w95) -> (w23:errorcluster)
      n380 = Obtain Queue(name (unnamed)="Continuous Send", element data type=Cont_Send_States_Brass."Run" ("State"), error in (no error)=w23) -> (queue out=w46:refnum<queue>, error out=w45:errorcluster)  [unwired: 2 in, 1 out]
      n381 = Obtain Queue(name (unnamed)="ERD Loop", element data type=T21 {"Data"=variant, "State"=enum."Read ERDs"} ("Data"), error in (no error)=w23) -> (queue out=w103:refnum<queue>, error out=w102:errorcluster)  [unwired: 2 in, 1 out]
      n382 = Obtain Queue(name (unnamed)="GEA2", element data type=T19 {"Data"=variant, "State"=enum."Add to Log"} ("Data"), error in (no error)=w23) -> (queue out=w112:refnum<queue>, error out=w111:errorcluster)  [unwired: 2 in, 1 out]
      n383 = Obtain Queue(name (unnamed)="DAQ", element data type=DAQ_States_Brass."Wait for Init" ("States"), error in (no error)=w23) -> (queue out=w98:refnum<queue>, error out=w99:errorcluster)  [unwired: 2 in, 1 out]
      n384 = Release Queue(queue=w46, error in (no error)=w45) -> (error out=w44:errorcluster)  [unwired: 1 in, 2 out]
      n385 = Release Queue(queue=w103, error in (no error)=w102) -> (error out=w91:errorcluster)  [unwired: 1 in, 2 out]
      n386 = Release Queue(queue=w112, error in (no error)=w111) -> (error out=w92:errorcluster)  [unwired: 1 in, 2 out]
      n387 = Release Queue(queue=w98, error in (no error)=w99) -> (error out=w93:errorcluster)  [unwired: 1 in, 2 out]
      n388 = Merge Errors(w44, w91, w92, w93) -> (w90:errorcluster)
      n389 = call "Error_Control_Brass.vi"("Command (Handle Errors)"=Error_Command_Brass."Report Errors", "Error In"=w90) -> ("Error Out"=w83:errorcluster)  [unwired: 13 in]
    }
    frame Error {
    }
  }
  n390 = call <vilib>:"Simple Error Handler.vi"("error in (no error)"=w2) -> ("error out"=→"Error Out":errorcluster)  [unwired: 4 in, 4 out]
